vi "WS1050 16 DUT Reliability HD_Cycling Ver1.7.vi"() -> ()   [LabVIEW 2012]
uses:
  Type Defs/WSVCAP SHL I2C DUT Mask Mode Enum.ctl
  <vilib>/Utility/file.llb/Read From Spreadsheet File (DBL).vi
  SubVI/Agilent E363X Series/Agilent E363X Series.lvlib
  SubVI/keithley_2000/Keithley 2000/Keithley 2000.lvlib
  SubVI/2012_Keithley 24XX/Keithley 24XX.lvlib
panel:
  out "VISA resource name out":refnum<visa-resource-name>="GPIB0::3::INSTR"
  out "error out 2":errorcluster={"status"=TRUE, "code"=-63192, "source"="niLvFpga_Open_PXI-7813R.vi"}
  in  "Reg1_Bit Cntrl":string[](array[string])=["01", "02", "04", "08", "10", "20", "40", "80", "03", "06", "0C", "D8", "33", "66", "CC", "07", "0E", "1C", "38", "70", "E0", "0F", "1E", "3C", "78", "F0", "1F", "3E", "7C", "F8", "3F", "7E", "FC", "7F", "FE", "FD", "FB", "F7", "EF", "DF", "BF", "7F", "FC", "F9", "F3", "E7", "CF", "9F", "3F", "F8", "F1", "E3", "C7", "8F", "1F", "F0", "E1", "C3", "87", "0F", "E0", "C1", "83", "07", "C0", "81", "03", "AA", "55", "00"]
  out "date string":string="5/19/2014"
  out "PS1 Out":refnum<visa-resource-name>
  out "Ke2000 Out":refnum<visa-resource-name>="GPIB0::9::INSTR"
  in  "Tab Control":T1(tab)=enum."Data Output"
  in  "Serial Number":string[][](table)=[["DUT", "SN"], ["DUT1", "1"], ["DUT2", "2"], ["DUT3", "3"], ["DUT4", "4"], ["DUT5", "5"], ["DUT6", "6"], ["DUT7", "7"], ["DUT8", "8"], ["DUT9", "9"], ["DUT10", "10"], ["DUT11", "11"], ["DUT12", "12"], ["DUT13", "13"], ["DUT14", "14"], ["DUT15", "15"], ["DUT16", "16"]]
  out "AD7747 Values":string[][](table)
  in  "SPI Clock Rate (Hz)":dbl=5000000.0 caption="Cycle Speed" format="%.1p Hz"
  in  "Lot#":string="3T9BB"
  in  "Wafer#":string="25-EB"
  in  "File Name":string="CYC_3T9BB_25_EB_65C_40V_50DC_BRD3_141107_1"
  in  "TMN DC\\CAP Data Log File Path":path=path "C:/WS1050 16 DUT Data"
  in  "Test Program":string="WS1050 16 DUT Reliability HD_Cycling Ver1.7"
  out "Current Date":string="8/28/2014"
  out "Current Time":string="0950"
  in  "Start Date":string="4/24/2014"
  in  "Start Time":string="1542"
  in  "Comment":string="CYC65C40V"
  in  "OK Button":bool
  in  "Calibration":bool
  in  "Verify CP":bool
  in  "CP Setting":i32(ring) items=["CP OFF", "CP ON", "CP 35V", "CP 40V", "DVA ON", "DVA OFF", "REG1 ON", "REG1 OFF", "REG2 ON", "REG2 OFF", "REG3 ON", "REG3 OFF"]
  in  "Stop Calibration":bool
  in  "Set VDD":dbl=3.7 format="%.3g"
  in  "Command":string[](array[string])=["0702013B3B3B", "070201000000"]
  in  "SPI Clock Rate (Hz)":dbl=1000000.0 caption="Meas Speed" format="%.1p Hz"
  out "AR  Meas(Hz)":dbl
  in  "PS1 Source":refnum<visa-resource-name>="GPIB0::5::INSTR"
  in  "Ke2000":refnum<visa-resource-name>="GPIB0::9::INSTR"
  in  "CP to HD/Cycle":i32(ring)=1 items=["CP HDC 35V", "CP HDC 40.25V", "CP HDC 27.5V", "CP HDC 30.5V", "CP HDC 44V"]
  out "Simulate FPGA":bool
  out "Online":bool
  out "AR Cycling(Hz)":dbl=5000000.0
  in  "Ke2400":refnum<visa-resource-name>="GPIB0::3::INSTR"
  in  "Initialize AD7747":bool
  in  "DUT Mask Mode":T2=enum."All"
  in  "RFFE Slave Address":u8=7 caption="Slave Address" format="0x%02x"
  out "Activity Log":string="05/19/2014 -- 12:24:35.853::WSVCAP::APP::Application Started\n05/19/2014 -- 12:24:37.606::WSVCAP::WSVCAP SHL::WR I2C-REG:0x0A;MASK:0xFFFFFFFFFFFF;C1 DATA:22:22:22:22:22:22:22:22:22:22:22:22:22:22:22:22;C2 DATA:22:22:22:22:22:22:22:22:22:22:22:22:22:22:22:22;C3 DATA:22:22:22:22:22:22:22:22:22:22:22:22:22:22:22:22\r\n05/19/2014 -- 12:24:37.773::WSVCAP::WSVCAP SHL::WR I2C-ST:0,0,4,1\r\n05/19/2014 -- 12:24:37.903::WSVCAP::WSVCAP SHL::RD I2C-BYTES:4;ADD:0x00;MASK:0xFFFFFFFFFFFF\r\n05/19/2014 -- 12:24:38.045::WSVCAP::WSVCAP SHL::RD I2C:C1 DATA:2:2:2:2:2:2:2:2:2:2:2:2:2:2:2:2|A7:A9:AA:82:82:7F:82:81:82:81:83:82:81:82:82:81|46:36:BB:88:44:A3:E9:2B:32:20:ED:25:BB:3D:68:B|2C:6A:EB:A7:22:56:FE:CC:36:82:D7:B0:3B:48:F9:CC;C2 DATA:2:2:2:2:2:2:2:2:2:2:2:2:2:2:2:2|94:94:94:80:80:80:80:80:81:7E:7E:81:80:7E:80:80|47:33:15:82:62:B:E8:1C:D7:C3:7D:41:7C:B7:4C:2A|C4:B4:AE:8:1E:D1:4E:37:11:C0:6F:63:42:9D:63:B5;C3 DATA:2:2:2:2:2:2:2:2:2:2:2:2:2:2:2:2|95:95:95:81:81:7E:81:80:84:7D:80:83:81:7E:7F:80|AB:C4:14:B5:7B:52:DF:C9:79:5D:5F:30:99:31:1E:F4|6E:5C:F7:A8:C3:EB:7B:EF:33:92:89:77:4D:67:75:DD;STATUS:0:0:4:0\r\n05/19/2014 -- 12:24:38.046::WSVCAP::WSVCAP SHL::WR I2C-REG:0x0A;MASK:0xFFFFFFFFFFFF;C1 DATA:22:22:22:22:22:22:22:22:22:22:22:22:22:22:22:22;C2 DATA:22:22:22:22:22:22:22:22:22:22:22:22:22:22:22:22;C3 DATA:22:22:22:22:22:22:22:22:22:22:22:22:22:22:22:22\r\n05/19/2014 -- 12:24:38.089::WSVCAP::WSVCAP SHL::WR I2C-ST:0,0,4,1\r\n05/19/2014 -- 12:24:38.219::WSVCAP::WSVCAP SHL::RD I2C-BYTES:4;ADD:0x00;MASK:0xFFFFFFFFFFFF\r\n05/19/2014 -- 12:24:38.362::WSVCAP::WSVCAP SHL::RD I2C:C1 DATA:2:2:2:2:2:2:2:2:2:2:2:2:2:2:2:2|A7:AB:AA:82:82:82:83:83:82:82:82:82:7F:82:82:81|4B:32:96:83:3E:61:43:17:25:62:AB:4D:A2:40:2E:5|3C:76:2B:B4:EE:E4:A9:1A:AA:A:26:C7:21:2E:87:5B;C2 DATA:2:2:2:2:2:2:2:2:2:2:2:2:2:2:2:2|94:94:94:80:80:80:80:80:80:7F:80:81:80:80:7F:80|4A:32:19:7D:19:6C:79:46:61:7F:4B:B8:A5:30:F3:14|B4:70:A:8C:9C:DC:43:FA:1E:A:C6:21:A:A9:13:F3;C3 DATA:2:2:2:2:2:2:2:2:2:2:2:2:2:2:2:2|95:97:94:81:80:81:82:81:80:7E:81:84:7F:81:80:80|B2:32:D0:A7:9E:4C:AB:D4:EE:D9:F0:82:B7:91:7:FF|C1:91:B6:3D:D8:E:1B:4F:9F:6A:F1:6C:E7:3F:7:BA;STATUS:0:0:4:0\r\n05/19/2014 -- 12:24:38.364::WSVCAP::WSVCAP SHL::WR I2C-REG:0x0A;MASK:0xFFFFFFFFFFFF;C1 DATA:22:22:22:22:22:22:22:22:22:22:22:22:22:22:22:22;C2 DATA:22:22:22:22:22:22:22:22:22:22:22:22:22:22:22:22;C3 DATA:22:22:22:22:22:22:22:22:22:22:22:22:22:22:22:22\r\n05/19/2014 -- 12:24:38.406::WSVCAP::WSVCAP SHL::WR I2C-ST:0,0,4,1\r\n05/19/2014 -- 12:24:38.536::WSVCAP::WSVCAP SHL::RD I2C-BYTES:4;ADD:0x00;MASK:0xFFFFFFFFFFFF\r\n05/19/2014 -- 12:24:38.678::WSVCAP::WSVCAP SHL::RD I2C:C1 DATA:2:2:2:2:2:2:2:2:2:2:2:2:2:2:2:2|A7:A9:AB:82:82:81:82:82:82:82:82:82:82:82:82:81|46:71:4C:87:43:3D:7F:FC:25:4F:8E:54:97:3E:60:8C|AA:F4:1F:B5:CE:43:1F:36:9:87:9C:78:86:5:B6:8E;C2 DATA:2:2:2:2:2:2:2:2:2:2:2:2:2:2:2:2|94:94:94:80:7F:7F:80:80:80:80:80:81:80:80:80:80|49:36:18:7D:6E:C5:E4:3C:81:2E:41:D3:75:71:E3:72|E8:D3:E6:D1:E0:48:AE:D4:54:D:E8:8E:B4:41:68:4;C3 DATA:2:2:2:2:2:2:2:2:2:2:2:2:2:2:2:2|95:95:95:81:7F:7F:81:81:81:81:81:84:81:81:82:81|B3:F5:90:AB:82:69:7B:93:D0:77:E8:D5:E8:8C:84:E8|B9:AC:EE:2B:B6:71:8F:4A:74:31:56:BB:8A:B7:A0:C8;STATUS:0:0:4:0\r\n05/19/2014 -- 12:24:38.681::WSVCAP::WSVCAP SHL::WR I2C-REG:0x0A;MASK:0xFFFFFFFFFFFF;C1 DATA:22:22:22:22:22:22:22:22:22:22:22:22:22:22:22:22;C2 DATA:22:22:22:22:22:22:22:22:22:22:22:22:22:22:22:22;C3 DATA:22:22:22:22:22:22:22:22:22:22:22:22:22:22:22:22\r\n05/19/2014 -- 12:24:38.723::WSVCAP::WSVCAP SHL::WR I2C-ST:0,0,4,1\r\n05/19/2014 -- 12:24:38.854::WSVCAP::WSVCAP SHL::RD I2C-BYTES:4;ADD:0x00;MASK:0xFFFFFFFFFFFF\r\n05/19/2014 -- 12:24:38.996::WSVCAP::WSVCAP SHL::RD I2C:C1 DATA:2:2:2:2:2:2:2:2:2:2:2:2:2:2:2:2|A7:A9:AA:82:82:7F:83:81:82:81:84:82:7F:82:7F:82|43:FB:E:7F:3C:AD:35:35:26:A2:6C:21:4B:3D:8:6|63:9A:E1:F3:95:32:91:42:90:3C:78:1F:5C:D7:5F:D8;C2 DATA:2:2:2:2:2:2:2:2:2:2:2:2:2:2:2:2|94:94:94:80:80:80:80:80:81:80:7E:81:80:7E:7F:80|48:36:18:7F:5E:3D:69:83:DE:AE:A1:9E:31:AE:BB:96|15:A0:44:17:13:FD:CC:C8:6D:B2:EF:A7:C:C7:3B:F;C3 DATA:2:2:2:2:2:2:2:2:2:2:2:2:2:2:2:2|95:96:94:81:81:7E:82:80:84:80:80:84:7F:7E:7D:82|AD:3B:6D:A9:7C:57:9D:F5:7A:96:23:5C:36:2D:ED:5A|CD:46:DB:3B:C7:BD:70:60:33:B8:B:F7:63:A:51:4D;STATUS:0:0:4:0\r\n05/19/2014 -- 12:24:38.998::WSVCAP::WSVCAP SHL::WR I2C-REG:0x0A;MASK:0xFFFFFFFFFFFF;C1 DATA:22:22:22:22:22:22:22:22:22:22:22:22:22:22:22:22;C2 DATA:22:22:22:22:22:22:22:22:22:22:22:22:22:22:22:22;C3 DATA:22:22:22:22:22:22:22:22:22:22:22:22:22:22:22:22\r\n05/19/2014 -- 12:24:39.040::WSVCAP::WSVCAP SHL::WR I2C-ST:0,0,4,1\r\n05/19/2014 -- 12:24:39.170::WSVCAP::WSVCAP SHL::RD I2C-BYTES:4;ADD:0x00;MASK:0xFFFFFFFFFFFF\r\n05/19/2014 -- 12:24:39.311::WSVCAP::WSVCAP SHL::RD I2C:C1 DATA:2:2:2:2:2:2:2:2:2:2:2:2:2:2:2:2|A7:AA:AB:82:82:81:82:81:82:81:82:82:82:82:7F:82|44:F1:90:87:45:44:C8:2C:2C:F1:FC:1B:94:3B:3C:75|4A:49:95:19:99:73:64:3:23:24:F3:A2:5E:7F:C4:B6;C2 DATA:2:2:2:2:2:2:2:2:2:2:2:2:2:2:2:2|94:94:94:80:80:80:80:7F:80:80:7E:80:80:7E:7F:80|4C:36:17:7D:A8:9F:DE:C7:53:6D:8A:F4:41:A5:C6:E0|90:2E:24:C:D9:22:E4:76:3B:40:1D:53:33:B1:3E:4D;C3 DATA:2:2:2:2:2:2:2:2:2:2:2:2:2:2:2:2|95:97:95:81:81:7F:81:80:80:81:7F:82:81:7E:7D:82|AE:2B:A7:AB:CC:CD:A4:38:FD:17:80:F2:92:2D:45:C4|76:E5:D:B9:AD:B5:BA:8D:28:32:9E:42:B7:20:4A:D9;STATUS:0:0:4:0\r\n05/19/2014 -- 12:24:39.313::WSVCAP::WSVCAP SHL::WR I2C-REG:0x0A;MASK:0xFFFFFFFFFFFF;C1 DATA:22:22:22:22:22:22:22:22:22:22:22:22:22:22:22:22;C2 DATA:22:22:22:22:22:22:22:22:22:22:22:22:22:22:22:22;C3 DATA:22:22:22:22:22:22:22:22:22:22:22:22:22:22:22:22\r\n05/19/2014 -- 12:24:39.355::WSVCAP::WSVCAP SHL::WR I2C-ST:0,0,4,1\r\n05/19/2014 -- 12:24:39.486::WSVCAP::WSVCAP SHL::RD I2C-BYTES:4;ADD:0x00;MASK:0xFFFFFFFFFFFF\r\n05/19/2014 -- 12:24:39.628::WSVCAP::WSVCAP SHL::RD I2C:C1 DATA:2:2:2:2:2:2:2:2:2:2:2:2:2:2:2:2|A7:A9:AA:82:82:82:83:82:82:82:82:82:7F:82:7F:82|47:18:E4:87:3E:E7:6:65:25:92:37:38:A8:3E:89:85|7C:A7:7:2B:A3:7A:EC:EF:89:ED:F4:D3:D8:BC:3A:F5;C2 DATA:2:2:2:2:2:2:2:2:2:2:2:2:2:2:2:2|94:94:94:80:7F:80:80:7F:81:80:7E:80:80:80:81:80|49:37:17:80:76:25:6A:F8:DF:55:97:4D:B8:5B:2B:B1|13:E3:9A:3E:1A:2D:4F:B6:DB:E9:61:FA:8B:D6:9:CC;C3 DATA:2:2:2:2:2:2:2:2:2:2:2:2:2:2:2:2|95:95:95:81:7F:80:82:81:84:80:7F:81:80:81:7F:82|AF:93:3B:AF:5B:11:82:E4:7E:C3:2D:72:9:96:D9:A|DB:96:F2:10:5F:64:9A:C6:98:12:27:7D:10:D3:20:D9;STATUS:0:0:4:0\r\n05/19/2014 -- 12:24:40.132::WSVCAP::WSVCAP SHL::CLOSE\r\n"
  in  "C1 Cap DAC":u8=128 caption="B Data In" format="0x%02x"
  in  "C2 Cap DAC":u8=128 caption="B Data In" format="0x%02x"
  in  "C3 Cap DAC":u8=128 caption="B Data In" format="0x%02x"
  out "IDD Brd(uA)":string
  in  "CP to Meas":i32(ring)=1 items=["CP HDC 35V", "CP HDC 40.25V", "CP HDC 27.5V", "CP HDC 30.5V", "CP HDC 44V"]
  in  "25% DC":dbl[](array[numeric])=[1.7e-05, 5e-05] min=0.0 max=0.5 format="%#.0p s"
  in  "50% DC":dbl[](array[numeric])=[3.3e-05, 3.3e-05] min=0.0 max=0.5 format="%#.0p s"
  in  "75% DC":dbl[](array[numeric])=[5e-05, 1.7e-05] min=0.0 max=0.5 format="%#.0p s"
  in  "CP VPI":i32(ring) items=["CP HDC 35V", "CP HDC 40.25V", "CP HDC 27.5V", "CP HDC 30.5V", "CP HDC 44V"]
  in  "Real No. From\nLookup Table":bool
  in  "Control Panel":T3={"Verify Socket"=FALSE, "HD/CYC"=FALSE, "E-CAL"=FALSE, "DVA"=FALSE, "VPI"=TRUE, "VSA"=TRUE, "HS"=TRUE}
  out "Verify Socket":bool
  out "HD/CYC":bool
  out "E-CAL":bool
  out "DVA":bool
  out "VPI":bool
  out "VSA":bool
  out "HS":bool
  in  "Cmd to HD":string="070201383838"
  in  "% Duty Cycle":enum16{"75%_DC", "50%_DC", "25%_DC"}(ring)=enum."25%_DC"
  in  "Set Time (s)\nFor Verify Socket":u32=300
  in  "Freq(Hz)":string="12K"
  in  "Brd #":string="1"
  out "error out":errorcluster
  in  "error in (no error)":errorcluster
  in  "WS1050/51":bool=TRUE
  in  "Test Sequences":i32(ring) items=["C1_C2_C3", "C2_C1_C3", "C3_C2_C1"]
  out "40V_1":string[][](table)
  out "VPI C1":string[][](table)
  out "VPI C3":string[][](table)
  out "NOM IDD OFF(uA)":string
  out "40V_2":string[][](table)
  out "VPI C2":string[][](table)
  out "NOM IDD ON (uA)":string
  out "40V_3":string[][](table)
  out "Total Time":u64
  out "IDD Stdby(uA)":string="2.606990E+0"
  out "EFuse RB T0":string[](array[string])
  out "Current EFuse Read back":string[](array[string])
  in  "Set HD/Cycle \nto Complete":u64=50000000000
  out "No of HD/Cycle\nCompleted":u64
  out "Cycle Count":u64 min=1 max=4 step=1
  out "Loop \ncompleted":i32=1
  out "Previous Time":string="12:20:26 PM"
  out "STATUS":string="Idle...."
  out "IDD_HD/CYC (uA)":string="164.601255E+0"
  in  "stop During HD/Cycles":bool
  in  "stop":bool
  out "Total Delta 2(pF)":string[](array[string])
  out "Total Delta 1(pF)":string[](array[string])
  out "Total Delta 3(pF)":string[](array[string])
  out "% Delta C_T0":string[][](array[string])
  out "% Delta C":string[][](array[string])
  out "EFuse Readback Status":bool[](array[boolean])
  in  "DeltaC Target(pF)_50":dbl=7.375
  out "RB Reg for HD":string[](array[string])
  out "RB Reg for HD/Cycle":string[](array[string])
  in  "DeltaC Target(pF)_51":dbl=5.875
  out "VSA_V1":string[][](table)
  out "VSA_V2":string[][](table)
  out "VSA_V3":string[][](table)
  in  "VSA Voltage(V)":dbl[](array[numeric])=[-10.0, 0.0, 10.0]
  in  "DC_Temp":i32=65
  in  "HD/CYC Temp":i32=65
  in  "Time All ON (s)":u32=120
  in  "Time All OFF (s)":u32=120
  in  "HD_DC (Min)":u64=259200
  out "LPs Count":i32
  in  "X Repeat":i32=100
  out "No LPs to RP":i32
  out "Running Loops":i32=1
  out "TTime Completed":u64=2000
  in  "TTF Completed":u64=50000000000
  in  "HD RP(Min)":dbl=60.0
  in  "CYC RP (X1000)":dbl=10000.0
  out "Min Plot_1":dbl[][](graph) caption="(Y) Multi Plot 2"
  out "Min Plot_2":dbl[][](graph) caption="(Y) Multi Plot 2"
  out "Min Plot_3":dbl[][](graph) caption="(Y) Multi Plot 2"
  in  "Debug":bool
  in  "No of Rows\nFrom Spread Sheet":i32
  in  "Plot Delta Cmin":bool=TRUE
  in  "Plot":T4(ring)
  # "Company:  WiSpry Inc\n20 Fairbanks Ste 198 \nIrvine CA 92618\n\nAuthor:  Andy V Tran\nCreated:  11/24/2014\nLabVIEW 2012 Pro\nTest Program:  WS1050 \n16 DUT HD/Cycle ver1.7\n\n*******************************"
  # "Note for HD during Cycles Setup:\n\n1.  Set HD/Cycle to Completed = 4320 minutes = 72 hours \n(T0 24hrs HD, T2 48hrs HD_Duty Cycle);  Default Setting\n2.  Set Time to Start HD Duty Cycle = 1440 = 24 hours\n3.  Set Time All ON = 120s = 2 minutes\n4.  Set Time All OFF = 120s = 2 minutes\n5.  No of Loops to RP = 3600s/(Time ALL ON(s) + Time ALL + OFF(s))\n6.  X Repeat = X runs\n7.  Set TTF Completed = Repeat X item1 to Stop.\n8.  Stop Test, set TTF Completed = Total Time Completed.\n\nNote for Cycling:\n\n\n\nVersion 1.7 is the latest verision for WS1050 16 DUT test program.\n\n1.  Added Test Sequences"
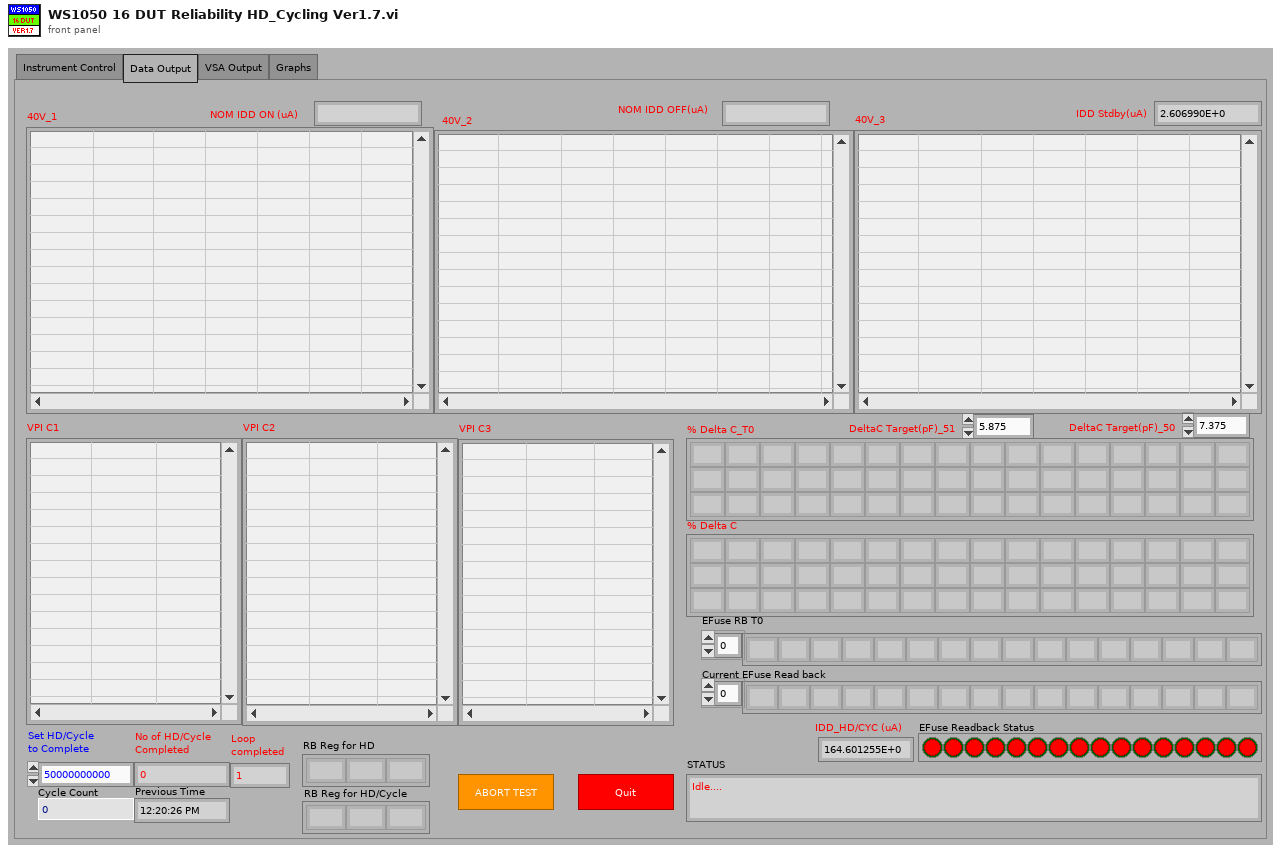
[diagram p1: front panel]
types:
  T1 = enum32{"Instrument Control", "Data Output", "VSA Output", "Graphs"}
  T2 = typedef "WSVCAP SHL I2C DUT Mask Mode Enum.ctl" = enum16{"Custom", "C1", "C2", "C3", "All"}
  T3 = cluster{"Verify Socket":bool, "HD/CYC":bool, "E-CAL":bool, "DVA":bool, "VPI":bool, "VSA":bool, "HS":bool}
  T4 = enum16{"DUT ALL", "DUT 01", "DUT 02", "DUT 03", "DUT 04", "DUT 05", "DUT 06", "DUT 07", "DUT 08", "DUT 09", "DUT 10", "DUT 11", "DUT 12", "DUT 13", "DUT 14", "DUT 15", "DUT 16"}
  T5 = typedef "WSVCAP SHL Core System Cluster.ctl" = cluster{"Settings":T6, "FPGA Resource":tag, "Online":bool, "I2C Wait Ticks":u32, "SPI Wait Ticks":u32, "RFFE Wait Ticks":u32}
  T6 = typedef "WSVCAP SHL I2C Settings Cluster.ctl" = cluster{"FPGA Resource Name":string, "I2C Slave Address":u8, "I2C Clock Rate (Hz)":dbl, "SPI Clock Rate (Hz)":dbl, "RFFE Slave Address":u8, "RFFE Clock Rate (Hz)":dbl, "Simulate FPGA":bool, "C1 Cap DAC Default":u8, "C2 Cap DAC Default":u8, "C3 Cap DAC Default":u8}
  T7 = enum16{"Idle...", "Voltage 1", "Voltage 2", "Voltage 3"}[]
  T8 = cluster{"Test Program ":string, "Comment":string, "Data Out":string, "Data Out":string, "Data Out":string, string, "Data Out":string, "Data Out":string, "string":string, "Freq(Hz)":string, "Brd #":string}
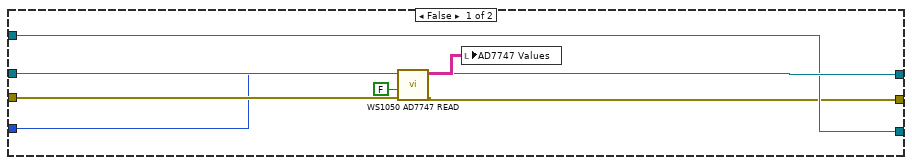
[diagram p9: hidden frame]
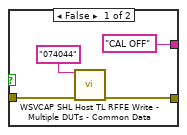
[diagram p10: hidden frame]
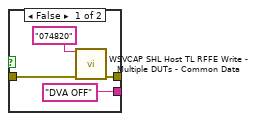
[diagram p11: hidden frame]
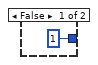
[diagram p12: hidden frame]
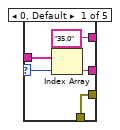
[diagram p13: hidden frame]
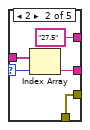
[diagram p14: hidden frame]
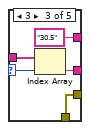
[diagram p15: hidden frame]
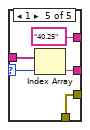
[diagram p16: hidden frame]
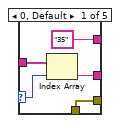
[diagram p17: hidden frame]
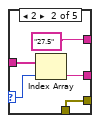
[diagram p18: hidden frame]
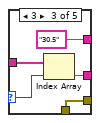
[diagram p19: hidden frame]
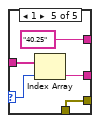
[diagram p20: hidden frame]
diagram:
  w18 = TRUE
  w24 = u16 0 items=["Off", "Moving Filter", "Repeating Filter"] ("Digital Filter (0: Off)")
  w25 = u16 7 items=["3.5 Digits"=4, "4.5 Digits"=5, "5.5 Digits"=6, "6.5 Digits"=7] ("Resolution (7: 6.5 digits)")
  n1 = case shown="True" w18 {
    tunnel: "error in (no error)" -> [w34 w35]
    tunnel: [w34 w42] -> w4
    frame False {
    }
    frame True {
      n2 = call "WSVCAP SHL Host TL Initialize.vi"("error in"=w35) -> ("error out"=w36:errorcluster)  [unwired: 13 in, 1 out]
      n3 = control-ref of="Activity Log"() -> (w38:refnum<vi>)
      n4 = call "ACT LG Activity Log Core.vi"("Display Ref"=w38, "Source"="WSVCAP", "Error In (no error)"=w36) -> ("Error Out"=w37:errorcluster)  [unwired: 11 in, 1 out]
      n5 = call "WSVCAP SHL Host TL Status Manager.vi"("error in"=w37) -> ("System Out"=w43:T5, "error out"=w42:errorcluster)  [unwired: 13 in]
      n6 = Unbundle By Name(w43) -> ("Online"=→"Online":bool, "Settings.Simulate FPGA"=→"Simulate FPGA":bool)
    }
  }
  n7 = case shown="True" TRUE {
    tunnel: w4 -> [w44 w49]
    tunnel: [w45 w48] -> w15
    tunnel: [w44 w47] -> w8
    tunnel: "Ke2400" -> [w45 w46]
    frame False {
    }
    frame True {
      n8 = VISA Write(VISA resource name=w46, write buffer="SOUR:FUNC VOLT;VOLT:MODE FIX;RANG 100;LEV 0.0;:SENS:FUNC \"CURR\";CURR:PROT 60E-3;RANG 100E-3;:OUTP ON", error in (no error)=w49) -> (VISA resource name out=w48:refnum<visa-resource-name>, error out=w47:errorcluster)  [unwired: 1 out]
    }
  }
  n9 = call "Initialize.vi"("VISA resource name"="Ke2000", "error in (no error)"=w4) -> ("VISA resource name out"=w27:refnum<visa-resource-name>, "error out"=w26:errorcluster)  [unwired: 16 in]
  n10 = call "Initialize.vi"("error in (no error)"=w4, "Reset? (T: Yes)"=FALSE, "ID Query? (T: Yes)"=TRUE, "VISA resource name"="PS1 Source") -> ("error out"=w3:errorcluster, "VISA resource name out"=w30:refnum<visa-resource-name>)  [unwired: 6 in]
  n11 = call "Configure DC Current.vi"("VISA resource name"=w27, "Resolution (7: 6.5 digits)"=w25, "error in (no error)"=w26, "Auto Range? (T: Auto)"=FALSE, "Digital Filter (0: Off)"=w24, "Custom Range (0 A)"=1.0) -> ("VISA resource name out"=w22:refnum<visa-resource-name>, "error out"=w5:errorcluster)  [unwired: 12 in]
  n12 = case shown="True" TRUE {
    tunnel: [_ w51] -> w33
    frame False {
    }
    frame True {
      n13 = call-poly <vilib>:"Read From Spreadsheet File.vi"("number of rows (all:-1)"=-1) -> ("all rows"=w51:dbl[][])  [unwired: 6 in, 4 out]
    }
  }
  n14 = Merge Errors(w8, w5, w3) -> (w16:errorcluster)
  n15 = while {
    tunnel: w16 -> [w73]
    tunnel: [w61] -> w12
    tunnel: w33 -> [w79]
    tunnel: w30 -> [w65]
    tunnel: w22 -> [w66]
    tunnel: [w77] -> w21
    tunnel: [w76] -> w20
    tunnel: [FALSE ("stop During HD/Cycles")] -> _
    tunnel: w15 -> [w72]
    tunnel: [w71] -> w13
    tunnel: [FALSE ("stop")] -> w6
    i -> [w74]
    stop <- w80 stop-if-true
    n16 = case shown="0" w74 {
      tunnel: w73 -> [w91 w93]
      tunnel: [w90 w93] -> w68
      tunnel: "RFFE Slave Address" -> [w88 _]
      frame 0 {
        w84 = dbl[][] []
        w83 = "" ("uA")
        w85 = string[][] []
        w86 = string[] [] ("EFuse Read back")
        w92 = u64 0 ("No of HD/Cycle\nCompleted")
        n17 = local write "RB Reg for HD/Cycle"(w86) -> ()
        n18 = local write "Current EFuse Read back"(w86) -> ()
        n19 = local write "EFuse RB T0"(w86) -> ()
        n20 = local write "No of HD/Cycle\nCompleted"(w92) -> ()
        n21 = local write "Cycle Count"(w92) -> ()
        n22 = local write "Total Delta 1(pF)"(w86) -> ()
        n23 = local write "Total Delta 2(pF)"(w86) -> ()
        n24 = local write "Total Delta 3(pF)"(w86) -> ()
        n25 = local write "VPI C2"(w85) -> ()
        n26 = local write "VSA_V3"(w85) -> ()
        n27 = local write "VSA_V1"(w85) -> ()
        n28 = local write "VSA_V2"(w85) -> ()
        n29 = local write "VPI C1"(w85) -> ()
        n30 = local write "VPI C3"(w85) -> ()
        n31 = local write "% Delta C"(w85) -> ()
        n32 = local write "% Delta C_T0"(w85) -> ()
        n33 = local write "40V_2"(w85) -> ()
        n34 = local write "40V_1"(w85) -> ()
        n35 = local write "40V_3"(w85) -> ()
        n36 = local write "NOM IDD OFF(uA)"(w83) -> ()
        n37 = local write "NOM IDD ON (uA)"(w83) -> ()
        n38 = local write "IDD Brd(uA)"(w83) -> ()
        n39 = local write "Min Plot_3"(w84) -> ()
        n40 = local write "Min Plot_1"(w84) -> ()
        n41 = local write "Min Plot_2"(w84) -> ()
        n42 = call "WSVCAP SHL Host TL RFFE Configure.vi"("RFFE Slave Address"=w88, "Clock Rate (Hz)"="SPI Clock Rate (Hz)", "error in"=w91) -> ("Actual Rate (Hz)"=→"AR  Meas(Hz)":dbl, "error out"=w90:errorcluster)  [unwired: 11 in]
      }
      frame 1, Default {
      }
    }
    n43 = while {
      tunnel: ["stop"] -> w70
      tunnel: w68 -> [w113]
      tunnel: [w104] -> w62
      tunnel: w65 -> [w111]
      tunnel: w66 -> [w106]
      tunnel: [w107] -> w64
      tunnel: [w105] -> w63
      tunnel: [w100] -> w59
      tunnel: [w99] -> w58
      tunnel: [w98] -> w57
      tunnel: [w97] -> w56
      tunnel: [w96] -> w55
      tunnel: [w95] -> w54
      tunnel: [w94] -> w53
      stop <- w120 stop-if-true
      # "Set Date & Time to Start Test"
      n44 = case shown="True" "Initialize AD7747" {
        tunnel: w113 -> [w129 w134]
        tunnel: [w129 w130] -> w112
        tunnel: w111 -> [w128 w132]
        tunnel: [w128 w131] -> w110
        frame False {
        }
        frame True {
          w135 = T7 [enum."Voltage 2", enum."Voltage 3", enum."Voltage 1"] items=["Idle...", "Voltage 1", "Voltage 2", "Voltage 3"]
          n45 = for {
            tunnel: w132 -> [w145]
            tunnel: w135 -> [w142] mode=indexing
            tunnel: [w141] -> w131
            shift-right: [w137] -> w133
            shift-left: w134 -> [w146]
            n46 = local read "Set VDD"() -> (w140:dbl)
            n47 = call "E3631A_Voltage Controller.vi"("VISA resource name"=w145, "I_VDD(A)"=0.2, "Channel Controller"=w142, "Voltage 1"=w140, "Voltage 2"=3.3, "error in (no error)"=w146, "Voltage 3"=-3.3) -> ("VISA resource name out"=w141:refnum<visa-resource-name>, "error out"=w136:errorcluster)  [unwired: 7 in]
            n48 = call "Delay T4.vi"("milliseconds to wait"=u32 100, "error in (no error)"=w136) -> ("error out"=w137:errorcluster)  [unwired: 9 in]
          }
          n49 = call "WS1050_AD7747_Init.vi"("error in"=w133) -> ("error out"=w130:errorcluster)  [unwired: 10 in]
        }
      }
      n50 = call "Time_stamp.vi"() -> ("date/time string"=w125:string, "date string"=w127:string)  [unwired: 2 in]
      "Current Date" <- w127
      "Current Time" <- w125
      n51 = Equal?(x=w127, y="Start Date") -> (x = y?=w123:bool)
      n52 = Equal?(x=w125, y="Start Time") -> (x = y?=w122:bool)
      n53 = And(x=w123, y=w122) -> (x .and. y?=w119:bool)
      n54 = Compound Arithmetic op=OR(w119, "OK Button", "stop") -> (w120:bool)
      n55 = case shown="True" "Calibration" {
        tunnel: w112 -> [w175 w193]
        tunnel: [w170 w190] -> w102
        tunnel: w110 -> [w174 w189]
        tunnel: "DUT Mask Mode" -> [w173 w185]
        tunnel: [w174 w184] -> w108
        tunnel: w106 -> [w172 w180]
        tunnel: [w172 w177] -> w105
        frame False {
          n56 = call "WS1050 AD7747 READ.vi"("error in"=w175, "Log (T)"=FALSE, "DUT Mask Mode (All)"=w173) -> ("error out"=w170:errorcluster, "AD7747 Values"=w176:string[][])  [unwired: 7 in]
          n57 = local write "AD7747 Values"(w176) -> ()
        }
        frame True {
          n58 = flat-sequence {
            tunnel: w193 -> [w202]
            tunnel: [w197] -> w192
            tunnel: w189 -> [w201]
            tunnel: [w200] -> w188
            tunnel: w185 -> [w199]
            tunnel: [w199] -> w186
            tunnel: w180 -> [w195]
            tunnel: [w194] -> w179
            tunnel: w192 -> [w226]
            tunnel: [w225] -> w191
            tunnel: w188 -> [w224]
            tunnel: [w224] -> w187
            tunnel: w186 -> [w223]
            tunnel: "C1 Cap DAC" -> [w219]
            tunnel: "C2 Cap DAC" -> [w218]
            tunnel: "C3 Cap DAC" -> [w217]
            tunnel: w179 -> [w216]
            tunnel: [w216] -> w178
            tunnel: w191 -> [w235]
            tunnel: [w238] -> w190
            tunnel: w187 -> [w237]
            tunnel: [w234] -> w184
            tunnel: w178 -> [w233]
            tunnel: [w233] -> w177
            frame #0 {
              w203 = T7 [enum."Voltage 2", enum."Voltage 3", enum."Voltage 1"] items=["Idle...", "Voltage 1", "Voltage 2", "Voltage 3"]
              n59 = for {
                tunnel: w201 -> [w214]
                tunnel: w203 -> [w211] mode=indexing
                tunnel: [w210] -> w200
                shift-right: [w208] -> w196
                shift-left: w202 -> [w215]
                n60 = local read "Set VDD"() -> (w205:dbl)
                n61 = call "E3631A_Voltage Controller.vi"("VISA resource name"=w214, "I_VDD(A)"=0.2, "Channel Controller"=w211, "Voltage 1"=w205, "Voltage 2"=3.3, "error in (no error)"=w215, "Voltage 3"=-3.3) -> ("VISA resource name out"=w210:refnum<visa-resource-name>, "error out"=w207:errorcluster)  [unwired: 7 in]
                n62 = call "Delay T4.vi"("milliseconds to wait"=u32 100, "error in (no error)"=w207) -> ("error out"=w208:errorcluster)  [unwired: 9 in]
              }
              n63 = One Button Dialog(message="Please verify all sockets should be empty...") -> ()  [unwired: 1 in, 1 out]
              n64 = call "Ke2000 Reading MilAmp.vi"("error in (no error)"=w196, "VISA resource name"=w195) -> ("error out"=w197:errorcluster, "uA"=→"IDD Brd(uA)":string, "VISA resource name out"=w194:refnum<visa-resource-name>)  [unwired: 7 in]
            }
            frame #1 {
              # "Calibration Multi-Sockets"
              n65 = call "WS1050 CAPDAC Setting.vi"("DUT Mask Mode (All)"=w223, "error in"=w226, "C3 Cap DAC"=w217, "C2 Cap DAC"=w218, "C1 Cap DAC"=w219) -> ("error out"=w221:errorcluster)  [unwired: 5 in, 1 out]
              n66 = call "WS1050 OFFSET CAL.vi"("error in"=w221, "OFFSET CAL"=TRUE ("Read?")) -> ("error out"=w220:errorcluster)  [unwired: 8 in, 1 out]
              n67 = while {
                tunnel: w220 -> [w232]
                tunnel: [w231] -> w225
                tunnel: w223 -> [w228]
                stop <- "Stop Calibration" stop-if-true
                n68 = call "WS1050 AD7747 READ.vi"("error in"=w232, "Log (T)"=FALSE, "DUT Mask Mode (All)"=w228) -> ("error out"=w231:errorcluster, "AD7747 Values"=→"AD7747 Values":string[][])  [unwired: 7 in]
              }
            }
            frame #2 {
              w236 = T7 [enum."Voltage 2", enum."Voltage 3", enum."Voltage 1"] items=["Idle...", "Voltage 1", "Voltage 2", "Voltage 3"]
              n69 = for {
                tunnel: w237 -> [w250]
                tunnel: w236 -> [w246] mode=indexing
                tunnel: [w245] -> w234
                shift-right: [w241] -> w238
                shift-left: w235 -> [w247]
                n70 = call "E3631A_Voltage Controller.vi"("VISA resource name"=w250, "I_VDD(A)"=0.2, "Channel Controller"=w246, "Voltage 1"=0.0, "Voltage 2"=3.3, "error in (no error)"=w247, "Voltage 3"=-3.3) -> ("VISA resource name out"=w245:refnum<visa-resource-name>, "error out"=w240:errorcluster)  [unwired: 7 in]
                n71 = call "Delay T4.vi"("milliseconds to wait"=u32 100, "error in (no error)"=w240) -> ("error out"=w241:errorcluster)  [unwired: 9 in]
              }
              n72 = One Button Dialog(message="Calibration Completed....") -> ()  [unwired: 1 in, 1 out]
            }
          }
        }
      }
      n73 = call "Control Panel.vi"("error in (no error)"=w102, "Control Panel"="Control Panel") -> ("error out"=w101:errorcluster, "VPI"=w96:bool, "DVA"=w97:bool, "E-CAL"=w98:bool, "VSA"=w95:bool, "HD/CYC"=w99:bool, "HS"=w94:bool, "Verify Socket"=w100:bool)  [unwired: 2 in]
      "Verify Socket" <- w100
      "HS" <- w94
      "VSA" <- w95
      "VPI" <- w96
      "E-CAL" <- w98
      "HD/CYC" <- w99
      "DVA" <- w97
      n74 = case shown="True" "Verify CP" {
        tunnel: [w147 w150] -> w104
        tunnel: w108 -> [w148 w155]
        tunnel: [w148 w153] -> w107
        tunnel: w101 -> [w147 w152]
        frame False {
        }
        frame True {
          w156 = T7 [enum."Voltage 2", enum."Voltage 3", enum."Voltage 1"] items=["Idle...", "Voltage 1", "Voltage 2", "Voltage 3"]
          # "Verify CP"
          n75 = for {
            tunnel: w155 -> [w168]
            tunnel: w156 -> [w165] mode=indexing
            shift-right: [w162] -> w154
            shift-left: w152 -> [w169]
            tunnel: [w160] -> w153
            n76 = local read "Set VDD"() -> (w164:dbl)
            n77 = call "E3631A_Voltage Controller.vi"("VISA resource name"=w168, "Channel Controller"=w165, "Voltage 1"=w164, "Voltage 2"=3.3, "error in (no error)"=w169, "Voltage 3"=-3.3) -> ("VISA resource name out"=w160:refnum<visa-resource-name>, "error out"=w163:errorcluster)  [unwired: 8 in]
            n78 = call "Delay T4.vi"("milliseconds to wait"=u32 100, "error in (no error)"=w163) -> ("error out"=w162:errorcluster)  [unwired: 9 in]
          }
          n79 = Index Array(array=string[] ["074000", "074040", "07476F", "074776", "074800", "074820", "07413B", "074100", "07423B", "074200", "07433B", "074300"], index="CP Setting") -> (element=w157:string)
          n80 = call "WSVCAP SHL Host TL RFFE Write - Multiple DUTs - Common Data.vi"("Data Out"=w157, "error in"=w154) -> ("error out"=w151:errorcluster)  [unwired: 13 in]
          n81 = call "Delay T4.vi"("milliseconds to wait"=u32 10, "error in (no error)"=w151) -> ("error out"=w150:errorcluster)  [unwired: 9 in]
        }
      }
      n82 = Wait Until Next ms Multiple(millisecond multiple=u32 100) -> ()  [unwired: 1 out]
    }
    n83 = case shown="False" w70 {
      tunnel: w62 -> [w306 w1818]
      tunnel: [w290 w1818] -> w61
      tunnel: w79 -> [w307 _]
      tunnel: w64 -> [w305 w1816]
      tunnel: w63 -> [w296 w1817]
      tunnel: [w303 w1817] -> w77
      tunnel: [w300 w1816] -> w76
      tunnel: w72 -> [w293 w1815]
      tunnel: [w289 w1815] -> w71
      tunnel: "RFFE Slave Address" -> [w284 _]
      tunnel: [FALSE ("stop During HD/Cycles") FALSE ("stop During HD/Cycles")] -> w60
      tunnel: w59 -> [w257 _]
      tunnel: w58 -> [w256 _]
      tunnel: w57 -> [w255 _]
      tunnel: w56 -> [w254 _]
      tunnel: w55 -> [w253 _]
      tunnel: w54 -> [w252 _]
      tunnel: w53 -> [w251 _]
      frame False {
        w285 = u64 0 ("Total Completed")
        w263 = u32 100 ("milliseconds to wait")
        w302 = T7 [enum."Voltage 2", enum."Voltage 3", enum."Voltage 1"] items=["Idle...", "Voltage 1", "Voltage 2", "Voltage 3"]
        w304 = T7 [enum."Voltage 2", enum."Voltage 3", enum."Voltage 1"] items=["Idle...", "Voltage 1", "Voltage 2", "Voltage 3"]
        # "DVA"
        # "Verify Socket"
        # "E-CAL"
        # "VSA"
        # "VPI"
        # "HS"
        # "DVA"
        # "HD/CYC"
        n84 = for {
          tunnel: w306 -> [w1813]
          tunnel: w305 -> [w1812]
          tunnel: w304 -> [w1809] mode=indexing
          tunnel: [w1804] -> w298
          tunnel: [w1808] -> w288
          n85 = local read "Set VDD"() -> (w1807:dbl)
          n86 = call "E3631A_Voltage Controller.vi"("VISA resource name"=w1812, "I_VDD(A)"=0.2, "Channel Controller"=w1809, "Voltage 1"=w1807, "Voltage 2"=3.3, "error in (no error)"=w1813, "Voltage 3"=-3.3) -> ("VISA resource name out"=w1808:refnum<visa-resource-name>, "error out"=w1805:errorcluster)  [unwired: 7 in]
          n87 = call "Delay T4.vi"("milliseconds to wait"=u32 100, "error in (no error)"=w1805) -> ("error out"=w1804:errorcluster)  [unwired: 9 in]
        }
        n88 = local write "TTime Completed"(w285) -> ()
        n89 = local write "Total Time"(w285) -> ()
        n90 = call "WSVCAP SHL Host TL RFFE Write - Multiple DUTs - Common Data.vi"("Data Out"="074000", "error in"=w298) -> ("error out"=w299:errorcluster)  [unwired: 13 in]
        n91 = local read "IDD Brd(uA)"() -> (w272:string)
        n92 = call "Delay T4.vi"("milliseconds to wait"=w263, "error in (no error)"=w299) -> ("error out"=w297:errorcluster)  [unwired: 9 in]
        n93 = Number To Fractional String(number="Set VDD", precision (6)=i16 2) -> (F-format string=w278:string)  [unwired: 2 in]
        n94 = call "Ke2000 Reading MilAmp.vi"("error in (no error)"=w297, "VISA resource name"=w296) -> ("error out"=w274:errorcluster, "uA"=w276:string, "VISA resource name out"=w295:refnum<visa-resource-name>)  [unwired: 7 in]
        n95 = call "Substration.vi"("error in (no error)"=w274, "Input2"=w272, "Input1"=w276) -> ("error out"=w273:errorcluster, "In1 - In2"=w275:string)  [unwired: 7 in]
        "IDD Stdby(uA)" <- w275
        n96 = call "WSVCAP SHL Host TL RFFE Write - Multiple DUTs - Common Data.vi"("Data Out"="074040", "error in"=w273) -> ("error out"=w258:errorcluster)  [unwired: 13 in]
        n97 = call "Delay T4.vi"("milliseconds to wait"=w263, "error in (no error)"=w258) -> ("error out"=w282:errorcluster)  [unwired: 9 in]
        n98 = case shown="True" w254 {
          tunnel: w282 -> [w329 w330]
          tunnel: [w328 w331] -> w280
          tunnel: ["DVA OFF" ("Data Out") "DVA ON" ("Data Out")] -> w281
          frame False {
            n99 = call "WSVCAP SHL Host TL RFFE Write - Multiple DUTs - Common Data.vi"("Data Out"="074820", "error in"=w329) -> ("error out"=w328:errorcluster)  [unwired: 13 in]
          }
          frame True {
            n100 = call "WSVCAP SHL Host TL RFFE Write - Multiple DUTs - Common Data.vi"("Data Out"="074800", "error in"=w330) -> ("error out"=w331:errorcluster)  [unwired: 13 in]
          }
        }
        n101 = for {
          N: 16 -> [_]
          tunnel: "Serial Number" -> [w312]
          tunnel: [w310] -> w260 mode=indexing
          i -> [w309]
          n102 = Increment(x=w309) -> (x+1=w308:i32)
          n103 = Index Array(array=w312, index (row)=w308, index (col)=1 ("disabled index (col)")) -> (element=w310:string)
        }
        n104 = case shown="True" w256 {
          tunnel: [1 ("X Repeat") w335] -> w287
          frame False {
          }
          frame True {
            n105 = local read "X Repeat"() -> (w335:i32)
          }
        }
        n106 = Not(x=w251) -> (.not. x?=w259:bool)
        n107 = call "Delay T4.vi"("milliseconds to wait"=w263, "error in (no error)"=w280) -> ("error out"=w267:errorcluster)  [unwired: 9 in]
        n108 = case shown="True" w255 {
          tunnel: w267 -> [w316 w318]
          tunnel: [w313 w317] -> w266
          tunnel: ["CAL OFF" ("Data Out") "CAL ON" ("Data Out")] -> w268
          frame False {
            n109 = call "WSVCAP SHL Host TL RFFE Write - Multiple DUTs - Common Data.vi"("Data Out"="074044", "error in"=w316) -> ("error out"=w313:errorcluster)  [unwired: 13 in]
          }
          frame True {
            n110 = for {
              tunnel: string[] ["074920", "074900"] -> [w325] mode=indexing
              tunnel: w318 -> [w322]
              tunnel: [w321] -> w317
              n111 = call "WSVCAP SHL Host TL RFFE Write - Multiple DUTs - Common Data.vi"("Data Out"=w325, "error in"=w322) -> ("error out"=w324:errorcluster)  [unwired: 13 in]
              n112 = call "Delay T4.vi"("milliseconds to wait"=u32 10, "error in (no error)"=w324) -> ("error out"=w321:errorcluster)  [unwired: 9 in]
            }
          }
        }
        n113 = for {
          N: w287 -> [_]
          tunnel: w307 -> [w372]
          tunnel: [w368] -> w303
          tunnel: [w367] -> w301
          tunnel: w275 -> [w366]
          tunnel: w295 -> [w365]
          tunnel: "TMN DC\\CAP Data Log File Path" -> [w364]
          tunnel: w293 -> [w362]
          tunnel: [w361] -> w291
          tunnel: w288 -> [w360]
          shift-right: [w355] -> _
          shift-left: u64 0 -> [w357]
          tunnel: w256 -> [w354]
          tunnel: w284 -> [w349]
          tunnel: w284 -> [w348]
          tunnel: w281 -> [w347]
          tunnel: w278 -> [w346]
          tunnel: [w345] -> w271
          tunnel: w268 -> [w344]
          tunnel: w266 -> [w343]
          tunnel: w254 -> [w342]
          tunnel: w257 -> [w340]
          tunnel: w253 -> [w339]
          tunnel: w259 -> [w338]
          tunnel: w252 -> [w337]
          tunnel: w260 -> [w336]
          i -> [w353]
          stop <- w341 stop-if-true
          n114 = while {
            tunnel: w372 -> [w592]
            tunnel: w364 -> [w603]
            tunnel: "Lot#" -> [w602]
            tunnel: "Wafer#" -> [w601]
            tunnel: w336 -> [w600]
            tunnel: "Test Program" -> [w599]
            tunnel: w336 -> [w598]
            tunnel: "Comment" -> [w597]
            tunnel: "Lot#" -> [w596]
            tunnel: "Wafer#" -> [w595]
            tunnel: w365 -> [w591]
            tunnel: [w594] -> w368
            tunnel: [w584] -> w367
            tunnel: w366 -> [w590]
            tunnel: w362 -> [w587]
            tunnel: [w586] -> w361
            tunnel: w360 -> [w585]
            tunnel: [w491] -> w351
            tunnel: w353 -> [w529]
            tunnel: [w520] -> w355
            tunnel: w357 -> [w519]
            shift-right: [w518] -> _
            shift-left: u64 0 -> [w412]
            tunnel: [w517] -> w350
            tunnel: w354 -> [w515]
            tunnel: w349 -> [w490]
            tunnel: w348 -> [w488]
            tunnel: w347 -> [w436]
            tunnel: w346 -> [w434]
            tunnel: [w409] -> w345
            tunnel: w344 -> [w416]
            tunnel: w343 -> [w415]
            tunnel: w342 -> [w414]
            tunnel: w340 -> [w406]
            tunnel: w339 -> [w405]
            tunnel: w338 -> [w400]
            tunnel: w337 -> [w394]
            i -> [w516]
            stop <- w530 stop-if-true
            n115 = case shown="4" "CP to HD/Cycle" {
              selector: "CP to HD/Cycle" -> [w607 w612 w617 w622 w626]
              tunnel: string[] ["07476F", "074776", "074765", "074769", "07477B"] -> [w608 w613 w618 w623 w628]
              tunnel: [w606 w611 w616 w621 w627] -> w431
              tunnel: ["35.0" ("Data Out") "27.5" ("Data Out") "30.5" ("Data Out") "44.0" ("Data Out") "40.25" ("Data Out")] -> w430
              tunnel: [w604 w609 w614 w619 w624] -> w429
              tunnel: w415 -> [w604 w609 w614 w619 w624]
              frame 0, Default {
                n116 = Index Array(array=w608, index=w607) -> (element=w606:string)
              }
              frame 2 {
                n117 = Index Array(array=w613, index=w612) -> (element=w611:string)
              }
              frame 3 {
                n118 = Index Array(array=w618, index=w617) -> (element=w616:string)
              }
              frame 4 {
                n119 = Index Array(array=w623, index=w622) -> (element=w621:string)
              }
              frame 1 {
                n120 = Index Array(array=w628, index=w626) -> (element=w627:string)
              }
            }
            n121 = flat-sequence {
              tunnel: [w693] -> w583
              tunnel: [w638] -> w582
              tunnel: w592 -> [w691]
              tunnel: [w690] -> w581
              tunnel: w591 -> [w667]
              tunnel: w590 -> [w689]
              tunnel: [w689] -> w580
              tunnel: [w632] -> w579
              tunnel: [w635] -> w578
              tunnel: w429 -> [w680]
              tunnel: [w647] -> w577
              tunnel: w585 -> [w687]
              tunnel: [w655] -> w584
              tunnel: w529 -> [w685]
              tunnel: w516 -> [w657]
              tunnel: [w657] -> w526
              tunnel: w516 -> [w684]
              tunnel: w515 -> [w682]
              tunnel: [w681] -> w514
              tunnel: [w643] -> w509
              tunnel: [w642] -> w508
              tunnel: [w641] -> w507
              tunnel: [w646] -> w497
              tunnel: [w644] -> w496
              tunnel: w490 -> [w679]
              tunnel: [w679] -> w489
              tunnel: w488 -> [w678]
              tunnel: [w645] -> w475
              tunnel: [w640] -> w449
              tunnel: [w677] -> w437
              tunnel: w431 -> [w675]
              tunnel: [w659] -> w428
              tunnel: [w658] -> w420
              tunnel: w406 -> [w651]
              tunnel: w405 -> [w650]
              tunnel: [w650] -> w404
              tunnel: w400 -> [w649]
              tunnel: [w649] -> w399
              tunnel: w394 -> [w648]
              tunnel: [w648] -> w393
              tunnel: ["WS1050/51"] -> w386
              tunnel: ["Test Sequences"] -> w376
              tunnel: "Real No. From\nLookup Table" -> [w629]
              tunnel: w583 -> [w1016]
              tunnel: [w1012] -> w487
              tunnel: w582 -> [w1015]
              tunnel: w581 -> [w1022]
              tunnel: [w1022] -> w486
              tunnel: w580 -> [w1021]
              tunnel: w579 -> [w1014]
              tunnel: w578 -> [w1013]
              tunnel: [w999] -> w485
              tunnel: [w1021] -> w484
              tunnel: [w1014] -> w483
              tunnel: [w1013] -> w482
              tunnel: w577 -> [w1019]
              tunnel: w526 -> [w1018]
              tunnel: [w1018] -> w481
              tunnel: w514 -> [w1017]
              tunnel: [w1017] -> w480
              tunnel: [w1015] -> w479
              tunnel: w509 -> [w1010]
              tunnel: w508 -> [w1004]
              tunnel: w507 -> [w1002]
              tunnel: [w1007] -> w478
              tunnel: w497 -> [w1009]
              tunnel: w496 -> [w1007]
              tunnel: [w1000] -> w477
              tunnel: w489 -> [w1008]
              tunnel: [w1005] -> w476
              tunnel: w475 -> [w1005]
              tunnel: [w1004] -> w474
              tunnel: w449 -> [w1003]
              tunnel: [w1003] -> w448
              tunnel: [w1002] -> w446
              tunnel: w437 -> [w1006]
              tunnel: [w1001] -> w421
              tunnel: w420 -> [w1001]
              tunnel: w404 -> [w998]
              tunnel: [w998] -> w403
              tunnel: w399 -> [w997]
              tunnel: [w997] -> w398
              tunnel: w393 -> [w996]
              tunnel: [w996] -> w392
              tunnel: w386 -> [w992]
              tunnel: [w992] -> w385
              tunnel: w376 -> [w991]
              tunnel: [w991] -> w375
              tunnel: w487 -> [w1126]
              tunnel: [w1125] -> w473
              tunnel: w486 -> [w1139]
              tunnel: [w1139] -> w470
              tunnel: w485 -> [w1138]
              tunnel: [w1138] -> w468
              tunnel: w484 -> [w1137]
              tunnel: [w1137] -> w466
              tunnel: w483 -> [w1136]
              tunnel: [w1136] -> w464
              tunnel: w482 -> [w1135]
              tunnel: [w1135] -> w462
              tunnel: w481 -> [w1134]
              tunnel: [w1134] -> w460
              tunnel: w480 -> [w1133]
              tunnel: [w1133] -> w458
              tunnel: w479 -> [w1132]
              tunnel: [w1132] -> w456
              tunnel: w478 -> [w1131]
              tunnel: [w1131] -> w454
              tunnel: [w1120] -> w452
              tunnel: w477 -> [w1119]
              tunnel: w476 -> [w1129]
              tunnel: w474 -> [w1127]
              tunnel: w448 -> [w1124]
              tunnel: [w1124] -> w447
              tunnel: w446 -> [w1123]
              tunnel: [w1123] -> w445
              tunnel: [w1121] -> w444
              tunnel: [w1122] -> w422
              tunnel: w421 -> [w1122]
              tunnel: w403 -> [w1118]
              tunnel: [w1118] -> w402
              tunnel: w398 -> [w1117]
              tunnel: [w1117] -> w397
              tunnel: w392 -> [w1116]
              tunnel: [w1116] -> w391
              tunnel: w385 -> [w1115]
              tunnel: [w1115] -> w384
              tunnel: w375 -> [w1114]
              tunnel: [w1114] -> w374
              tunnel: w473 -> [w1212]
              tunnel: [w1211] -> w472
              tunnel: [w1207] -> w471
              tunnel: w470 -> [w1224]
              tunnel: [w1224] -> w469
              tunnel: w468 -> [w1223]
              tunnel: [w1223] -> w467
              tunnel: w466 -> [w1222]
              tunnel: [w1222] -> w465
              tunnel: w464 -> [w1221]
              tunnel: [w1221] -> w463
              tunnel: w462 -> [w1220]
              tunnel: [w1220] -> w461
              tunnel: w460 -> [w1219]
              tunnel: [w1219] -> w459
              tunnel: w458 -> [w1218]
              tunnel: [w1218] -> w457
              tunnel: w456 -> [w1217]
              tunnel: [w1217] -> w455
              tunnel: w454 -> [w1216]
              tunnel: [w1216] -> w453
              tunnel: w452 -> [w1215]
              tunnel: [w1215] -> w451
              tunnel: [w1205] -> w450
              tunnel: w447 -> [w1214]
              tunnel: w445 -> [w1213]
              tunnel: w444 -> [w1206]
              tunnel: [w1210] -> w435
              tunnel: [w1209] -> w423
              tunnel: w422 -> [w1209]
              tunnel: w414 -> [w1208]
              tunnel: [w1208] -> w413
              tunnel: w402 -> [w1204]
              tunnel: [w1204] -> w401
              tunnel: w397 -> [w1203]
              tunnel: [w1203] -> w396
              tunnel: w391 -> [w1202]
              tunnel: [w1202] -> w390
              tunnel: w384 -> [w1201]
              tunnel: [w1201] -> w383
              tunnel: [w1201] -> w381
              tunnel: [w1201] -> w380
              tunnel: w374 -> [w1200]
              tunnel: [w1351] -> w576
              tunnel: [w1317] -> w575
              tunnel: w472 -> [w1355]
              tunnel: w471 -> [w1331]
              tunnel: [w1340] -> w574
              tunnel: [w1331] -> w573
              tunnel: [w1354] -> w572
              tunnel: [w1353] -> w571
              tunnel: w469 -> [w1352]
              tunnel: [w1352] -> w570
              tunnel: w467 -> [w1340]
              tunnel: w465 -> [w1350]
              tunnel: [w1350] -> w569
              tunnel: w463 -> [w1346]
              tunnel: [w1346] -> w568
              tunnel: w461 -> [w1345]
              tunnel: [w1345] -> w567
              tunnel: w459 -> [w1341]
              tunnel: [w1341] -> w525
              tunnel: w457 -> [w1349]
              tunnel: [w1349] -> w513
              tunnel: w455 -> [w1348]
              tunnel: [w1347] -> w510
              tunnel: w453 -> [w1343]
              tunnel: w451 -> [w1339]
              tunnel: [w1344] -> w506
              tunnel: [w1342] -> w505
              tunnel: [w1339] -> w500
              tunnel: w450 -> [w1338]
              tunnel: [w1325] -> w495
              tunnel: [w1324] -> w494
              tunnel: [w1323] -> w493
              tunnel: w435 -> [w1337]
              tunnel: [w1322] -> w424
              tunnel: w423 -> [w1322]
              tunnel: [w1321] -> w419
              tunnel: w413 -> [w1320]
              tunnel: w401 -> [w1315]
              tunnel: w396 -> [w1314]
              tunnel: [w1314] -> w395
              tunnel: w390 -> [w1313]
              tunnel: [w1313] -> w389
              tunnel: w383 -> [w1303]
              tunnel: [w1303] -> w382
              tunnel: w381 -> [w1302]
              tunnel: w380 -> [w1301]
              tunnel: w576 -> [w1568]
              tunnel: [w1568] -> w566
              tunnel: [w1553] -> w565
              tunnel: [w1567] -> w564
              tunnel: w575 -> [w1566]
              tunnel: w574 -> [w1565]
              tunnel: w573 -> [w1564]
              tunnel: [w1565] -> w563
              tunnel: [w1564] -> w562
              tunnel: w572 -> [w1563]
              tunnel: [w1563] -> w561
              tunnel: w571 -> [w1562]
              tunnel: [w1562] -> w560
              tunnel: w570 -> [w1561]
              tunnel: [w1561] -> w559
              tunnel: w569 -> [w1560]
              tunnel: [w1560] -> w558
              tunnel: w568 -> [w1559]
              tunnel: [w1559] -> w557
              tunnel: w567 -> [w1558]
              tunnel: [w1558] -> w556
              tunnel: w587 -> [w1557]
              tunnel: [w1555] -> w555
              tunnel: [w1535] -> w554
              tunnel: [w1536] -> w553
              tunnel: [w1534] -> w552
              tunnel: w525 -> [w1551]
              tunnel: [w1551] -> w524
              tunnel: w513 -> [w1550]
              tunnel: [w1550] -> w512
              tunnel: w510 -> [w1567]
              tunnel: w506 -> [w1548]
              tunnel: w505 -> [w1549]
              tunnel: [w1549] -> w504
              tunnel: [w1548] -> w502
              tunnel: w500 -> [w1547]
              tunnel: [w1547] -> w499
              tunnel: w495 -> [w1533]
              tunnel: w494 -> [w1532]
              tunnel: w493 -> [w1531]
              tunnel: [w1528] -> w492
              tunnel: [w1533] -> w443
              tunnel: [w1532] -> w441
              tunnel: [w1531] -> w439
              tunnel: [w1530] -> w425
              tunnel: w424 -> [w1530]
              tunnel: w419 -> [w1529]
              tunnel: [w1529] -> w418
              tunnel: w395 -> [w1528]
              tunnel: w389 -> [w1527]
              tunnel: w382 -> [w1526]
              tunnel: [w1526] -> w379
              tunnel: w566 -> [w1654]
              tunnel: [w1654] -> w551
              tunnel: w565 -> [w1678]
              tunnel: [w1677] -> w550
              tunnel: w603 -> [w1679]
              tunnel: w602 -> [w1676]
              tunnel: w601 -> [w1675]
              tunnel: w600 -> [w1674]
              tunnel: [w1673] -> w549
              tunnel: w564 -> [w1667]
              tunnel: [w1667] -> w548
              tunnel: w563 -> [w1672]
              tunnel: w562 -> [w1671]
              tunnel: [w1672] -> w547
              tunnel: [w1671] -> w546
              tunnel: [w1662] -> w545
              tunnel: w561 -> [w1670]
              tunnel: [w1670] -> w544
              tunnel: w560 -> [w1669]
              tunnel: [w1669] -> w543
              tunnel: w559 -> [w1666]
              tunnel: [w1668] -> w542
              tunnel: w412 -> [w1665]
              tunnel: [w1664] -> w541
              tunnel: [w1652] -> w540
              tunnel: w558 -> [w1663]
              tunnel: w557 -> [w1661]
              tunnel: w556 -> [w1660]
              tunnel: "File Name" -> [w1659]
              tunnel: w555 -> [w1658]
              tunnel: [w1658] -> w539
              tunnel: w554 -> [w1657]
              tunnel: [w1657] -> w538
              tunnel: [w1656] -> w537
              tunnel: w553 -> [w1656]
              tunnel: w552 -> [w1655]
              tunnel: [w1655] -> w536
              tunnel: [w1650] -> w527
              tunnel: w524 -> [w1651]
              tunnel: [w1651] -> w522
              tunnel: w519 -> [w1649]
              tunnel: w512 -> [w1648]
              tunnel: [w1648] -> w511
              tunnel: w504 -> [w1647]
              tunnel: [w1647] -> w503
              tunnel: w502 -> [w1646]
              tunnel: [w1646] -> w501
              tunnel: w499 -> [w1645]
              tunnel: [w1645] -> w498
              tunnel: w492 -> [w1644]
              tunnel: w443 -> [w1643]
              tunnel: [w1643] -> w442
              tunnel: w441 -> [w1642]
              tunnel: [w1642] -> w440
              tunnel: w439 -> [w1641]
              tunnel: [w1641] -> w438
              tunnel: w428 -> [w1640]
              tunnel: [w1640] -> w427
              tunnel: [w1639] -> w426
              tunnel: w425 -> [w1639]
              tunnel: w418 -> [w1638]
              tunnel: [w1638] -> w417
              tunnel: ["Freq(Hz)"] -> w388
              tunnel: ["Brd #"] -> w387
              tunnel: w379 -> [w1635]
              tunnel: [w1635] -> w378
              tunnel: w551 -> [w1750]
              tunnel: w550 -> [w1749]
              tunnel: w603 -> [w1711]
              tunnel: w599 -> [w1744]
              tunnel: w598 -> [w1747]
              tunnel: w597 -> [w1743]
              tunnel: w596 -> [w1746]
              tunnel: w595 -> [w1742]
              tunnel: w549 -> [w1745]
              tunnel: [w1750] -> w532
              tunnel: [w1748] -> w533
              tunnel: w548 -> [w1740]
              tunnel: [w1740] -> w534
              tunnel: w547 -> [w1739]
              tunnel: w546 -> [w1724]
              tunnel: w545 -> [w1738]
              tunnel: w544 -> [w1737]
              tunnel: w543 -> [w1726]
              tunnel: [w1734] -> w535
              tunnel: w542 -> [w1736]
              tunnel: w541 -> [w1735]
              tunnel: w540 -> [w1734]
              tunnel: "File Name" -> [w1704]
              tunnel: w539 -> [w1733]
              tunnel: [w1733] -> w531
              tunnel: w538 -> [w1732]
              tunnel: w537 -> [w1731]
              tunnel: w536 -> [w1730]
              tunnel: [w1729] -> w528
              tunnel: w527 -> [w1729]
              tunnel: [w1707] -> w523
              tunnel: w522 -> [w1707]
              tunnel: w511 -> [w1728]
              tunnel: w503 -> [w1727]
              tunnel: w501 -> [w1725]
              tunnel: w498 -> [w1723]
              tunnel: w442 -> [w1722]
              tunnel: w440 -> [w1721]
              tunnel: w438 -> [w1720]
              tunnel: w436 -> [w1719]
              tunnel: w416 -> [w1717]
              tunnel: w430 -> [w1716]
              tunnel: w434 -> [w1715]
              tunnel: w427 -> [w1714]
              tunnel: w426 -> [w1713]
              tunnel: w417 -> [w1712]
              tunnel: [w1709] -> w411
              tunnel: [w1700] -> w407
              tunnel: w388 -> [w1699]
              tunnel: w387 -> [w1698]
              tunnel: w378 -> [w1697]
              tunnel: [w1697] -> w377
              tunnel: [w1772] -> w593
              tunnel: [w1773] -> w594
              tunnel: [w1774] -> w491
              tunnel: w535 -> [w1765]
              tunnel: w534 -> [w1773]
              tunnel: w533 -> [w1760]
              tunnel: w532 -> [w1774]
              tunnel: w531 -> [w1767]
              tunnel: [w1767] -> w586
              tunnel: [w1764] -> w520
              tunnel: w528 -> [w1764]
              tunnel: w523 -> [w1766]
              tunnel: [w1766] -> w521
              tunnel: [w1765] -> w518
              tunnel: [w1763] -> w517
              tunnel: [w1759] -> w408
              tunnel: w411 -> [w1758]
              tunnel: w407 -> [w1756]
              tunnel: w377 -> [w1755]
              frame #0 {
                n122 = call "WSVCAP SHL Host TL RFFE Write - Multiple DUTs - Common Data.vi"("Data Out"=w675, "error in"=w680) -> ("error out"=w653:errorcluster)  [unwired: 13 in]
                n123 = Index Array(array=w691, index (row)=w684, index (col)=0 ("disabled index (col)")) -> (element=w683:dbl)
                n124 = for {
                  tunnel: string[] ["0760", "0767", "0768"] -> [w738] mode=indexing
                  tunnel: [w734] -> w664 mode=indexing
                  tunnel: w653 -> [w732]
                  tunnel: [w731] -> w656
                  i -> [w737]
                  n125 = call "Delay T4.vi"("milliseconds to wait"=u32 10, "error in (no error)"=w732) -> ("error out"=w739:errorcluster)  [unwired: 9 in]
                  n126 = call "WSVCAP SHL Host TL RFFE Read - Multiple DUTs - Common Data.vi"("Data Out"=w738, "error in"=w739) -> ("RFFE Data In"=w736:string[], "error out"=w731:errorcluster)  [unwired: 12 in]
                  n127 = Index Array(array=w736, index=w737) -> (element=w733:string)
                  n128 = String Subset(string=w733, offset (0)=0) -> (substring=w734:string)  [unwired: 1 in]
                }
                "RB Reg for HD/Cycle" <- w664
                n129 = call "Delay T4.vi"("milliseconds to wait"=u32 100, "error in (no error)"=w656) -> ("error out"=w670:errorcluster)  [unwired: 9 in]
                n130 = local read "IDD Brd(uA)"() -> (w674:string)
                n131 = call "Ke2000 Reading MilAmp.vi"("error in (no error)"=w670, "VISA resource name"=w667) -> ("error out"=w672:errorcluster, "uA"=w673:string, "VISA resource name out"=w666:refnum<visa-resource-name>)  [unwired: 7 in]
                n132 = call "Substration.vi"("error in (no error)"=w672, "Input2"=w674, "Input1"=w673) -> ("error out"=w669:errorcluster, "In1 - In2"=→"IDD_HD/CYC (uA)":string)  [unwired: 7 in]
                n133 = case shown="False" w682 {
                  tunnel: [w772 w878] -> w693
                  tunnel: [w773 w863] -> w688
                  tunnel: [w771 w880] -> w690
                  tunnel: w669 -> [w767 w867]
                  tunnel: w687 -> [w763 w879]
                  tunnel: [w763 w879] -> w655
                  tunnel: w685 -> [_ w869]
                  tunnel: w683 -> [w764 w864]
                  tunnel: [w769 w865] -> w681
                  tunnel: w657 -> [w750 w861]
                  tunnel: w678 -> [w766 _]
                  tunnel: [w760 "100" ("Data Out")] -> w659
                  tunnel: w651 -> [w748 _]
                  tunnel: w629 -> [w747 w854]
                  frame False {
                    # "Cycles in 1s"
                    n134 = case shown="False" w747 {
                      tunnel: w767 -> [w779 w785]
                      tunnel: w764 -> [w778 w784]
                      tunnel: [w777 w785] -> w762
                      tunnel: w750 -> [w776 _]
                      tunnel: [w775 w784] -> w757
                      tunnel: [u64 1000 ("y") u64 1 ("y")] -> w751
                      frame False {
                        n135 = case shown="8, Default" w776 {
                          tunnel: w778 -> [w781 _]
                          tunnel: [w781 "CYC RP (X1000)"] -> w775
                          tunnel: [w780 w782] -> w777
                          tunnel: w779 -> [w780 w782]
                          frame 0..7 {
                          }
                          frame 8, Default {
                          }
                        }
                      }
                      frame True {
                        # "Read real number\nfrom lookup table"
                      }
                    }
                    n136 = call "WSVCAP SHL Host TL RFFE Configure.vi"("RFFE Slave Address"=w766, "Clock Rate (Hz)"="SPI Clock Rate (Hz)", "error in"=w762) -> ("Actual Rate (Hz)"=→"AR Cycling(Hz)":dbl, "error out"=w758:errorcluster)  [unwired: 11 in]
                    n137 = case shown="\"50%_DC\", Default" "% Duty Cycle" {
                      tunnel: ["75% DC" "50% DC" "25% DC"] -> w755
                      tunnel: ["75" ("Data Out") "50" ("Data Out") "25" ("Data Out")] -> w760
                      tunnel: [w787 w790 w793] -> w759
                      tunnel: w758 -> [w787 w790 w793]
                      frame "75%_DC" {
                      }
                      frame "50%_DC", Default {
                      }
                      frame "25%_DC" {
                      }
                    }
                    n138 = Array Max & Min(array=w755) -> (max value=w754:dbl)  [unwired: 3 out]
                    n139 = Divide(x=1.0, y=w754) -> (x/y=w753:dbl)
                    n140 = To Unsigned Quad Integer(1:w753) -> (0:w752:u64)
                    n141 = Not(x=w748) -> (.not. x?=w749:bool)
                    n142 = case shown="False" w749 {
                      tunnel: [w797 w819] -> w773
                      tunnel: [w800 w818] -> w772
                      tunnel: [u64 1 w817] -> w771
                      tunnel: w759 -> [w798 w816]
                      tunnel: w757 -> [_ w815]
                      tunnel: w755 -> [_ w812]
                      tunnel: w752 -> [_ w811]
                      tunnel: w751 -> [_ w810]
                      tunnel: w750 -> [w796 _]
                      frame False {
                        n143 = case shown="1, Default" w796 {
                          tunnel: w798 -> [w801 w803]
                          tunnel: [w801 w802] -> w797
                          frame 0 {
                          }
                          frame 1, Default {
                            n144 = flat-sequence {
                              tunnel: "Set Time (s)\nFor Verify Socket" -> [w809]
                              tunnel: w803 -> [w806]
                              tunnel: [w806] -> w802
                              frame #0 {
                                n145 = Multiply(x=w809, y=u32 1000) -> (x*y=w808:u32)
                                n146 = Wait (ms)(milliseconds to wait=w808) -> ()  [unwired: 1 out]
                                n147 = local write "STATUS"("Verify Sockets waiting times..." ("STATUS")) -> ()
                              }
                            }
                          }
                        }
                        n148 = local read "stop During HD/Cycles"() -> (w800:bool)
                      }
                      frame True {
                        n149 = while {
                          tunnel: w815 -> [w839]
                          tunnel: [w826] -> w819
                          tunnel: [w831] -> w818
                          tunnel: w816 -> [w837]
                          tunnel: [w825] -> w817
                          tunnel: "Command" -> [w836]
                          tunnel: w812 -> [w835]
                          tunnel: w811 -> [w822]
                          tunnel: w810 -> [w820]
                          i -> [w834]
                          stop <- w830 stop-if-true
                          # "At least 1 second before target"
                          # "Remaining Cycles"
                          # "Target Cycles"
                          # "Cycles in 1s"
                          n150 = To Unsigned Quad Integer(1:w839) -> (0:w838:u64)
                          n151 = case shown="0" w834 {
                            tunnel: [w846 w848] -> w828
                            tunnel: w837 -> [w847 w848]
                            tunnel: w836 -> [w845 _]
                            tunnel: w835 -> [w844 _]
                            frame 0 {
                              n152 = call "WSVCAP SHL Host TL RFFE Write Cycle - Multiple DUTs - Common Data1.vi"("Data Out (Cycle Commands)"=w845, "Post Command Delay"=w844, "error in"=w847) -> ("error out"=w846:errorcluster)  [unwired: 12 in]
                            }
                            frame 1, Default {
                            }
                          }
                          n153 = Multiply(x=w838, y=w820) -> (x*y=w825:u64)
                          n154 = call "WSVCAP SHL Host TL SPI_RFFE Query Cycle Count.vi"("error in"=w828) -> ("Cycle Count"=w824:u64, "error out"=w833:errorcluster)  [unwired: 13 in]
                          "Cycle Count" <- w824
                          n155 = Subtract(x=w825, y=w824) -> (x-y=w823:u64)
                          n156 = Greater Or Equal?(x=w824, y=w825) -> (x >= y?=w832:bool)
                          n157 = local read "stop During HD/Cycles"() -> (w831:bool)
                          n158 = Greater?(x=w823, y=w822) -> (0:w821:bool)
                          n159 = case shown="True" w832 {
                            tunnel: [w850 w853] -> w827
                            tunnel: w833 -> [w850 w852]
                            tunnel: [FALSE TRUE] -> w829
                            frame False {
                            }
                            frame True {
                              n160 = call "WSVCAP SHL Host TL RFFE Stop Write Cycle.vi"("error in"=w852) -> ("error out"=w853:errorcluster)  [unwired: 14 in]
                            }
                          }
                          n161 = Or(x=w829, y=w831) -> (x .or. y?=w830:bool)
                          n162 = case shown="True" w821 {
                            tunnel: w827 -> [w840 w843]
                            tunnel: [w840 w842] -> w826
                            frame False {
                            }
                            frame True {
                              n163 = call "MISC Wait with Data Flow.vi"("Error In (no error)"=w843, "Wait Time (500ms)"=u32 50) -> ("Error Out"=w842:errorcluster)  [unwired: 7 in, 2 out]
                            }
                          }
                        }
                        n164 = local write "STATUS"("Parts are Cycling...." ("STATUS")) -> ()
                      }
                    }
                    n165 = local read "HD/CYC Temp"() -> (w768:i32)
                    n166 = Number To Engineering String(4:w768) -> (0:w769:string)  [unwired: 3 in]
                  }
                  frame True {
                    n167 = case shown="False" w854 {
                      tunnel: w869 -> [w886 _]
                      tunnel: [w885 w898] -> w868
                      tunnel: w867 -> [w884 w899]
                      tunnel: [w883 w899] -> w866
                      tunnel: w864 -> [w882 w898]
                      tunnel: w861 -> [w881 _]
                      frame False {
                        n168 = case shown="0" w886 {
                          tunnel: [w889 w896] -> w885
                          tunnel: w884 -> [w891 w897]
                          tunnel: [w890 w897] -> w883
                          tunnel: w882 -> [w888 _]
                          tunnel: w881 -> [w887 _]
                          frame 0 {
                            n169 = case shown="15, Default" w887 {
                              tunnel: [w892 "HD RP(Min)"] -> w889
                              tunnel: w891 -> [w893 w895]
                              tunnel: [w893 w895] -> w890
                              tunnel: w888 -> [w892 _]
                              frame 0..14 {
                              }
                              frame 15, Default {
                              }
                            }
                          }
                          frame 1, Default {
                            n170 = local read "HD RP(Min)"() -> (w896:dbl)
                          }
                        }
                      }
                      frame True {
                      }
                    }
                    n171 = flat-sequence {
                      tunnel: [w973] -> w874
                      tunnel: w866 -> [w979]
                      frame #0 {
                        n172 = call "WSVCAP SHL Host TL RFFE Write - Multiple DUTs - Common Data.vi"("Data Out"="Cmd to HD", "error in"=w979) -> ("error out"=w978:errorcluster)  [unwired: 13 in]
                        n173 = call "Delay T4.vi"("milliseconds to wait"=u32 50, "error in (no error)"=w978) -> ("error out"=w975:errorcluster)  [unwired: 9 in]
                        n174 = for {
                          tunnel: string[] ["0761", "0762", "0763"] -> [w990] mode=indexing
                          tunnel: [w986] -> w974 mode=indexing
                          shift-right: [w983] -> w973
                          shift-left: w975 -> [w989]
                          i -> [w988]
                          n175 = call "WSVCAP SHL Host TL RFFE Read - Multiple DUTs - Common Data.vi"("Data Out"=w990, "error in"=w989) -> ("RFFE Data In"=w985:string[], "error out"=w982:errorcluster)  [unwired: 12 in]
                          n176 = Index Array(array=w985, index=w988) -> (element=w984:string)
                          n177 = call "Delay T4.vi"("milliseconds to wait"=u32 10, "error in (no error)"=w982) -> ("error out"=w983:errorcluster)  [unwired: 9 in]
                          n178 = String Subset(string=w984, offset (0)=0) -> (substring=w986:string)  [unwired: 1 in]
                        }
                        "RB Reg for HD" <- w974
                      }
                    }
                    n179 = local read "No of HD/Cycle\nCompleted"() -> (w870:u64)
                    n180 = Greater?(x="HD_DC (Min)", y=w870) -> (0:w871:bool)
                    n181 = case shown="True" w871 {
                      tunnel: [_ w906] -> w876
                      tunnel: [w901 w905] -> w875
                      tunnel: w874 -> [w901 w904]
                      tunnel: w868 -> [w900 w903]
                      tunnel: [w900 w902] -> w873
                      frame False {
                      }
                      frame True {
                        n182 = flat-sequence {
                          tunnel: [w911] -> w906
                          tunnel: [w910] -> w905
                          tunnel: w904 -> [w909]
                          tunnel: w903 -> [w907]
                          tunnel: [w907] -> w902
                          frame #0 {
                            # "HD"
                            n183 = Multiply(x=1000.0, y=w907) -> (x*y=w914:dbl)
                            n184 = Multiply(x=60.0, y=w914) -> (x*y=w912:dbl)
                            n185 = local write "STATUS"("Parts are Holding Down..." ("STATUS")) -> ()
                            n186 = event shown="[0] Timeout" {
                              selector: _ -> [_ _]
                              dyn-events: _ -> [_ _]
                              timeout: w912 -> [_ _]
                              tunnel: ["stop During HD/Cycles" TRUE ("stop During HD/Cycles")] -> w911
                              tunnel: w909 -> [w916 w918]
                              tunnel: [w916 w918] -> w910
                              event Timeout {
                                n187 = event-data() -> ()  [unwired: 1 in, 2 out]
                              }
                              event "stop During HD/Cycles": Value Change {
                                n188 = event-data() -> ()  [unwired: 1 in, 2 out]
                              }
                            }
                          }
                        }
                      }
                    }
                    n189 = Greater Or Equal?(x=w870, y="HD_DC (Min)") -> (x >= y?=w877:bool)
                    n190 = To Unsigned Quad Integer(1:w868) -> (0:w880:u64)
                    n191 = Add(x="Time All OFF (s)", y="Time All ON (s)") -> (x+y=w856:u32)
                    n192 = To Double Precision Float(number=w856) -> (double precision float=w855:dbl)
                    n193 = Divide(x=w855, y=60.0) -> (x/y=w857:dbl)
                    n194 = case shown="False" w877 {
                      tunnel: [w922 w935] -> w878
                      tunnel: [w923 w927] -> w863
                      tunnel: w875 -> [w923 w934]
                      tunnel: w876 -> [w922 w933]
                      tunnel: w873 -> [_ w932]
                      tunnel: [w921 w930] -> w865
                      tunnel: w857 -> [_ w924]
                      frame False {
                        n195 = Number To Engineering String(4:"HD/CYC Temp") -> (0:w921:string)  [unwired: 3 in]
                      }
                      frame True {
                        n196 = Divide(x=w932, y=w924) -> (x/y=w931:dbl)
                        n197 = call "WSVCAP SHL Host TL RFFE Write - Multiple DUTs - Common Data.vi"("Data Out"="070201000000", "error in"=w934) -> ("error out"=w937:errorcluster)  [unwired: 13 in]
                        n198 = Round To Nearest(number=w931) -> (nearest integer value=w926:dbl)
                        n199 = call "Delay T4.vi"("milliseconds to wait"=u32 50, "error in (no error)"=w937) -> ("error out"=w928:errorcluster)  [unwired: 9 in]
                        n200 = To Long Integer(number=w926) -> (32bit integer=w925:i32)
                        "No LPs to RP" <- w925
                        n201 = for {
                          N: w925 -> [_]
                          tunnel: w933 -> [w952]
                          tunnel: [w951] -> w935
                          tunnel: w928 -> [w940]
                          tunnel: [w939] -> w927
                          i -> [w950]
                          stop <- w951 stop-if-true
                          n202 = Increment(x=w950) -> (x+1=→"LPs Count":i32)
                          n203 = call "WSVCAP SHL Host TL RFFE Write - Multiple DUTs - Common Data.vi"("Data Out"="074776", "error in"=w940) -> ("error out"=w958:errorcluster)  [unwired: 13 in]
                          n204 = call "Delay T4.vi"("milliseconds to wait"=u32 1, "error in (no error)"=w958) -> ("error out"=w957:errorcluster)  [unwired: 9 in]
                          n205 = local read "CP to HD/Cycle"() -> (w942:i32)
                          n206 = call "WSVCAP SHL Host TL RFFE Write - Multiple DUTs - Common Data.vi"("Data Out"="070201000000", "error in"=w943) -> ("error out"=w954:errorcluster)  [unwired: 13 in]
                          n207 = call "WSVCAP SHL Host TL RFFE Write - Multiple DUTs - Common Data.vi"("Data Out"="0702013B3B3B", "error in"=w957) -> ("error out"=w947:errorcluster)  [unwired: 13 in]
                          n208 = flat-sequence {
                            tunnel: w954 -> [w966]
                            tunnel: [w964] -> w939
                            frame #0 {
                              n209 = local read "Time All OFF (s)"() -> (w961:u32)
                              n210 = local write "STATUS"("Now HD OFF Time..." ("STATUS")) -> ()
                              n211 = Multiply(x=w961, y=u32 1000) -> (x*y=w963:u32)
                              n212 = call "Delay T4.vi"("milliseconds to wait"=w963, "error in (no error)"=w966) -> ("error out"=w964:errorcluster)  [unwired: 9 in]
                            }
                          }
                          n213 = call "Delay T4.vi"("milliseconds to wait"=u32 1, "error in (no error)"=w947) -> ("error out"=w945:errorcluster)  [unwired: 9 in]
                          n214 = Index Array(array=string[] ["07476F", "074776", "074765", "074769", "07477B"], index=w942) -> (element=w948:string)
                          n215 = call "WSVCAP SHL Host TL RFFE Write - Multiple DUTs - Common Data.vi"("Data Out"=w948, "error in"=w945) -> ("error out"=w944:errorcluster)  [unwired: 13 in]
                          n216 = flat-sequence {
                            tunnel: [w971] -> w943
                            tunnel: w944 -> [w967]
                            frame #0 {
                              n217 = local read "Time All ON (s)"() -> (w968:u32)
                              n218 = local write "STATUS"("Now HD ON Time..." ("STATUS")) -> ()
                              n219 = Multiply(x=w968, y=u32 1000) -> (x*y=w970:u32)
                              n220 = call "Delay T4.vi"("milliseconds to wait"=w970, "error in (no error)"=w967) -> ("error out"=w971:errorcluster)  [unwired: 9 in]
                            }
                          }
                          n221 = Unbundle By Name(w939) -> ("status"=w953:bool)
                          n222 = Or(x=w953, y=w952) -> (x .or. y?=w951:bool)
                        }
                        n223 = Number To Engineering String(4:"DC_Temp") -> (0:w930:string)  [unwired: 3 in]
                      }
                    }
                  }
                }
                n224 = case shown="4" "CP to Meas" {
                  selector: "CP to Meas" -> [w709 w714 w719 w724 w728]
                  tunnel: string[] ["07476F", "074776", "074765", "074769", "07477B"] -> [w710 w715 w720 w725 w730]
                  tunnel: [w708 w713 w718 w723 w729] -> w662
                  tunnel: [w707 w712 w717 w722 w727] -> w652
                  tunnel: w661 -> [w707 w712 w717 w722 w727]
                  tunnel: ["35" ("Data Out") "27.5" ("Data Out") "30.5" ("Data Out") "44.0" ("Data Out") "40.25" ("Data Out")] -> w658
                  frame 0, Default {
                    n225 = Index Array(array=w710, index=w709) -> (element=w708:string)
                  }
                  frame 2 {
                    n226 = Index Array(array=w715, index=w714) -> (element=w713:string)
                  }
                  frame 3 {
                    n227 = Index Array(array=w720, index=w719) -> (element=w718:string)
                  }
                  frame 4 {
                    n228 = Index Array(array=w725, index=w724) -> (element=w723:string)
                  }
                  frame 1 {
                    n229 = Index Array(array=w730, index=w728) -> (element=w729:string)
                  }
                }
                n230 = call "WSVCAP SHL Host TL RFFE Write - Multiple DUTs - Common Data.vi"("Data Out"=w662, "error in"=w652) -> ("error out"=w676:errorcluster)  [unwired: 13 in]
                n231 = flat-sequence {
                  tunnel: w688 -> [w746]
                  tunnel: [w746] -> w661
                  frame #0 {
                    w742 = "0" ("NOM IDD OFF(uA)")
                    w743 = string[] []
                    w744 = string[][] []
                    n232 = To Long Integer(number=0.0 ("No of Loops to RP")) -> (32bit integer=w741:i32)
                    n233 = local write "LPs Count"(w741) -> ()
                    n234 = local write "No LPs to RP"(w741) -> ()
                    n235 = local write "NOM IDD ON (uA)"(w742) -> ()
                    n236 = local write "Current EFuse Read back"(w743) -> ()
                    n237 = local write "RB Reg for HD"(w743) -> ()
                    n238 = local write "RB Reg for HD/Cycle"(w743) -> ()
                    n239 = local write "NOM IDD OFF(uA)"(w742) -> ()
                    n240 = local write "Total Delta 1(pF)"(w743) -> ()
                    n241 = local write "Total Delta 2(pF)"(w743) -> ()
                    n242 = local write "Total Delta 3(pF)"(w743) -> ()
                    n243 = local write "VSA_V3"(w744) -> ()
                    n244 = local write "VSA_V1"(w744) -> ()
                    n245 = local write "VSA_V2"(w744) -> ()
                    n246 = local write "VPI C1"(w744) -> ()
                    n247 = local write "VPI C2"(w744) -> ()
                    n248 = local write "VPI C3"(w744) -> ()
                    n249 = local write "% Delta C"(w744) -> ()
                    n250 = local write "40V_3"(w744) -> ()
                    n251 = local write "40V_2"(w744) -> ()
                    n252 = local write "40V_1"(w744) -> ()
                  }
                }
                n253 = call "Delay T4.vi"("milliseconds to wait"=u32 50, "error in (no error)"=w676) -> ("error out"=w654:errorcluster)  [unwired: 9 in]
                n254 = for {
                  tunnel: [w705] -> w633 mode=indexing
                  tunnel: w666 -> [w703]
                  tunnel: w654 -> [w702]
                  tunnel: [w696] -> w638
                  tunnel: string[] ["0702013B3B3B", "070201000000"] -> [w695] mode=indexing
                  tunnel: [w694] -> w631
                  n255 = call "WSVCAP SHL Host TL RFFE Write - Multiple DUTs - Common Data.vi"("Data Out"=w695, "error in"=w702) -> ("error out"=w699:errorcluster)  [unwired: 13 in]
                  n256 = call "Delay T4.vi"("milliseconds to wait"=u32 100, "error in (no error)"=w699) -> ("error out"=w700:errorcluster)  [unwired: 9 in]
                  n257 = local read "IDD Brd(uA)"() -> (w704:string)
                  n258 = call "Ke2000 Reading MilAmp.vi"("error in (no error)"=w700, "VISA resource name"=w703) -> ("error out"=w698:errorcluster, "uA"=w697:string, "VISA resource name out"=w696:refnum<visa-resource-name>)  [unwired: 7 in]
                  n259 = call "Substration.vi"("error in (no error)"=w698, "Input2"=w704, "Input1"=w697) -> ("error out"=w694:errorcluster, "In1 - In2"=w705:string)  [unwired: 7 in]
                }
                n260 = Index Array(array=w633, index=0) -> (element=w635:string)
                n261 = Index Array(array=w633, index=1) -> (element=w632:string)
                n262 = call "Multi Dut Cmd Setting.vi"("error in (no error)"=w631, "Test Seq"="Test Sequences", "WS1050/51"="WS1050/51") -> ("error out"=w647:errorcluster, "Cmd 3"=w641:string[], "Name 3"=w640:string[], "Name Header"=w644:string[], "Cmd 2"=w642:string[], "Name 2"=w645:string[], "Cmd 1"=w643:string[], "Name 1"=w646:string[])  [unwired: 1 in]
                n263 = local read "SPI Clock Rate (Hz)"() -> (w677:dbl)
              }
              frame #1 {
                n264 = call "WSVCAP SHL Host TL RFFE Configure.vi"("RFFE Slave Address"=w1008, "Clock Rate (Hz)"=w1006, "error in"=w1019) -> ("Actual Rate (Hz)"=w1020:dbl, "error out"=w994:errorcluster)  [unwired: 11 in]
                n265 = local write "AR  Meas(Hz)"(w1020) -> ()
                n266 = Array Size(array=w1009) -> (size(s)=w1023:i32)
                n267 = call "Delay T4.vi"("milliseconds to wait"=u32 10, "error in (no error)"=w994) -> ("error out"=w995:errorcluster)  [unwired: 9 in]
                n268 = case shown="2" w991 {
                  tunnel: w1023 -> [w1031 w1061 w1091]
                  tunnel: w1016 -> [w1030 w1060 w1090]
                  tunnel: [w1029 w1059 w1089] -> w1012
                  tunnel: [w1028 w1058 w1088] -> w1011
                  tunnel: w1010 -> [w1027 w1057 w1087]
                  tunnel: w1009 -> [w1026 w1056 w1086]
                  tunnel: [w1025 w1055 w1085] -> w1000
                  tunnel: w995 -> [w1024 w1054 w1084]
                  frame 0, Default {
                    n269 = for {
                      N: w1031 -> [_]
                      tunnel: w1027 -> [w1049]
                      tunnel: w1030 -> [w1047]
                      tunnel: [w1046] -> w1029
                      tunnel: [w1042] -> w1028 mode=indexing
                      tunnel: w1026 -> [w1044]
                      tunnel: w1024 -> [w1032]
                      tunnel: [w1034] -> w1025
                      i -> [w1041]
                      stop <- w1046 stop-if-true
                      n270 = Index Array(array=w1049, index=w1041) -> (element=w1045:string)
                      n271 = Index Array(array=w1044, index=w1041) -> (element=w1043:string)
                      n272 = local write "STATUS"(w1043) -> ()
                      n273 = call "WSVCAP SHL Host TL RFFE Write - Multiple DUTs - Common Data.vi"("Data Out"=w1045, "error in"=w1032) -> ("error out"=w1036:errorcluster)  [unwired: 13 in]
                      n274 = call "Delay T4.vi"("milliseconds to wait"=u32 10, "error in (no error)"=w1036) -> ("error out"=w1040:errorcluster)  [unwired: 9 in]
                      n275 = call "WS1050 AD7747 READ.vi"("error in"=w1040, "Log (T)"=FALSE, "DUT Mask Mode (All)"=WSVCAP_SHL_I2C_DUT_Mask_Mode_Enum."C1") -> ("error out"=w1038:errorcluster, "AD7747 Values"=w1039:string[][])  [unwired: 7 in]
                      n276 = for {
                        tunnel: w1039 -> [w1052] mode=indexing
                        tunnel: w1038 -> [w1053]
                        tunnel: [w1053] -> w1034
                        tunnel: [w1050] -> w1042 mode=indexing
                        n277 = Index Array(array=w1052, index=1) -> (element=w1050:string)
                      }
                      n278 = Unbundle By Name(w1034) -> ("status"=w1048:bool)
                      n279 = Or(x=w1048, y=w1047) -> (x .or. y?=w1046:bool)
                    }
                  }
                  frame 1 {
                    n280 = for {
                      N: w1061 -> [_]
                      tunnel: w1057 -> [w1079]
                      tunnel: w1060 -> [w1077]
                      tunnel: [w1076] -> w1059
                      tunnel: [w1072] -> w1058 mode=indexing
                      tunnel: w1056 -> [w1074]
                      tunnel: w1054 -> [w1062]
                      tunnel: [w1064] -> w1055
                      i -> [w1071]
                      stop <- w1076 stop-if-true
                      n281 = Index Array(array=w1079, index=w1071) -> (element=w1075:string)
                      n282 = Index Array(array=w1074, index=w1071) -> (element=w1073:string)
                      n283 = local write "STATUS"(w1073) -> ()
                      n284 = call "WSVCAP SHL Host TL RFFE Write - Multiple DUTs - Common Data.vi"("Data Out"=w1075, "error in"=w1062) -> ("error out"=w1066:errorcluster)  [unwired: 13 in]
                      n285 = call "Delay T4.vi"("milliseconds to wait"=u32 10, "error in (no error)"=w1066) -> ("error out"=w1070:errorcluster)  [unwired: 9 in]
                      n286 = call "WS1050 AD7747 READ.vi"("error in"=w1070, "Log (T)"=FALSE, "DUT Mask Mode (All)"=WSVCAP_SHL_I2C_DUT_Mask_Mode_Enum."C2") -> ("error out"=w1068:errorcluster, "AD7747 Values"=w1069:string[][])  [unwired: 7 in]
                      n287 = for {
                        tunnel: w1069 -> [w1082] mode=indexing
                        tunnel: w1068 -> [w1083]
                        tunnel: [w1083] -> w1064
                        tunnel: [w1080] -> w1072 mode=indexing
                        n288 = Index Array(array=w1082, index=3) -> (element=w1080:string)
                      }
                      n289 = Unbundle By Name(w1064) -> ("status"=w1078:bool)
                      n290 = Or(x=w1078, y=w1077) -> (x .or. y?=w1076:bool)
                    }
                  }
                  frame 2 {
                    n291 = for {
                      N: w1091 -> [_]
                      tunnel: w1087 -> [w1109]
                      tunnel: w1090 -> [w1107]
                      tunnel: [w1106] -> w1089
                      tunnel: [w1102] -> w1088 mode=indexing
                      tunnel: w1086 -> [w1104]
                      tunnel: w1084 -> [w1092]
                      tunnel: [w1094] -> w1085
                      i -> [w1101]
                      stop <- w1106 stop-if-true
                      n292 = Index Array(array=w1109, index=w1101) -> (element=w1105:string)
                      n293 = Index Array(array=w1104, index=w1101) -> (element=w1103:string)
                      n294 = local write "STATUS"(w1103) -> ()
                      n295 = call "WSVCAP SHL Host TL RFFE Write - Multiple DUTs - Common Data.vi"("Data Out"=w1105, "error in"=w1092) -> ("error out"=w1096:errorcluster)  [unwired: 13 in]
                      n296 = call "Delay T4.vi"("milliseconds to wait"=u32 10, "error in (no error)"=w1096) -> ("error out"=w1100:errorcluster)  [unwired: 9 in]
                      n297 = call "WS1050 AD7747 READ.vi"("error in"=w1100, "Log (T)"=FALSE, "DUT Mask Mode (All)"=WSVCAP_SHL_I2C_DUT_Mask_Mode_Enum."C3") -> ("error out"=w1098:errorcluster, "AD7747 Values"=w1099:string[][])  [unwired: 7 in]
                      n298 = for {
                        tunnel: w1099 -> [w1112] mode=indexing
                        tunnel: w1098 -> [w1113]
                        tunnel: [w1113] -> w1094
                        tunnel: [w1110] -> w1102 mode=indexing
                        n299 = Index Array(array=w1112, index=5) -> (element=w1110:string)
                      }
                      n300 = Unbundle By Name(w1094) -> ("status"=w1108:bool)
                      n301 = Or(x=w1108, y=w1107) -> (x .or. y?=w1106:bool)
                    }
                  }
                }
                n302 = Transpose 2D Array(2D array=w1011) -> (transposed array=w999:string[][])
                "40V_1" <- w999
                "NOM IDD ON (uA)" <- w1014
                "NOM IDD OFF(uA)" <- w1013
              }
              frame #2 {
                n303 = Array Size(array=w1129) -> (size(s)=w1130:i32)
                n304 = case shown="0, 2, Default" w1114 {
                  tunnel: w1130 -> [w1147 w1177]
                  tunnel: w1129 -> [w1146 w1176]
                  tunnel: [w1145 w1175] -> w1128
                  tunnel: w1127 -> [w1144 w1174]
                  tunnel: w1126 -> [w1143 w1173]
                  tunnel: [w1142 w1172] -> w1125
                  tunnel: [w1141 w1171] -> w1121
                  tunnel: w1119 -> [w1140 w1170]
                  frame 0, 2, Default {
                    n305 = for {
                      N: w1147 -> [_]
                      tunnel: w1144 -> [w1165]
                      tunnel: w1143 -> [w1163]
                      tunnel: [w1162] -> w1142
                      tunnel: [w1158] -> w1145 mode=indexing
                      tunnel: w1146 -> [w1160]
                      tunnel: w1140 -> [w1148]
                      tunnel: [w1150] -> w1141
                      i -> [w1157]
                      stop <- w1162 stop-if-true
                      n306 = Index Array(array=w1165, index=w1157) -> (element=w1161:string)
                      n307 = Index Array(array=w1160, index=w1157) -> (element=w1159:string)
                      n308 = call "WSVCAP SHL Host TL RFFE Write - Multiple DUTs - Common Data.vi"("Data Out"=w1161, "error in"=w1148) -> ("error out"=w1152:errorcluster)  [unwired: 13 in]
                      n309 = local write "STATUS"(w1159) -> ()
                      n310 = call "Delay T4.vi"("milliseconds to wait"=u32 10, "error in (no error)"=w1152) -> ("error out"=w1156:errorcluster)  [unwired: 9 in]
                      n311 = call "WS1050 AD7747 READ.vi"("error in"=w1156, "Log (T)"=FALSE, "DUT Mask Mode (All)"=WSVCAP_SHL_I2C_DUT_Mask_Mode_Enum."C2") -> ("error out"=w1154:errorcluster, "AD7747 Values"=w1155:string[][])  [unwired: 7 in]
                      n312 = for {
                        tunnel: w1155 -> [w1168] mode=indexing
                        tunnel: w1154 -> [w1169]
                        tunnel: [w1169] -> w1150
                        tunnel: [w1166] -> w1158 mode=indexing
                        n313 = Index Array(array=w1168, index=3) -> (element=w1166:string)
                      }
                      n314 = Unbundle By Name(w1150) -> ("status"=w1164:bool)
                      n315 = Or(x=w1164, y=w1163) -> (x .or. y?=w1162:bool)
                    }
                  }
                  frame 1 {
                    n316 = for {
                      N: w1177 -> [_]
                      tunnel: w1174 -> [w1195]
                      tunnel: w1173 -> [w1193]
                      tunnel: [w1192] -> w1172
                      tunnel: [w1188] -> w1175 mode=indexing
                      tunnel: w1176 -> [w1190]
                      tunnel: w1170 -> [w1178]
                      tunnel: [w1180] -> w1171
                      i -> [w1187]
                      stop <- w1192 stop-if-true
                      n317 = Index Array(array=w1195, index=w1187) -> (element=w1191:string)
                      n318 = Index Array(array=w1190, index=w1187) -> (element=w1189:string)
                      n319 = call "WSVCAP SHL Host TL RFFE Write - Multiple DUTs - Common Data.vi"("Data Out"=w1191, "error in"=w1178) -> ("error out"=w1182:errorcluster)  [unwired: 13 in]
                      n320 = local write "STATUS"(w1189) -> ()
                      n321 = call "Delay T4.vi"("milliseconds to wait"=u32 10, "error in (no error)"=w1182) -> ("error out"=w1186:errorcluster)  [unwired: 9 in]
                      n322 = call "WS1050 AD7747 READ.vi"("error in"=w1186, "Log (T)"=FALSE, "DUT Mask Mode (All)"=WSVCAP_SHL_I2C_DUT_Mask_Mode_Enum."C1") -> ("error out"=w1184:errorcluster, "AD7747 Values"=w1185:string[][])  [unwired: 7 in]
                      n323 = for {
                        tunnel: w1185 -> [w1198] mode=indexing
                        tunnel: w1184 -> [w1199]
                        tunnel: [w1199] -> w1180
                        tunnel: [w1196] -> w1188 mode=indexing
                        n324 = Index Array(array=w1198, index=1) -> (element=w1196:string)
                      }
                      n325 = Unbundle By Name(w1180) -> ("status"=w1194:bool)
                      n326 = Or(x=w1194, y=w1193) -> (x .or. y?=w1192:bool)
                    }
                  }
                }
                n327 = Transpose 2D Array(2D array=w1128) -> (transposed array=w1120:string[][])
                "40V_2" <- w1120
              }
              frame #3 {
                n328 = case shown="True" w1201 {
                  tunnel: w1214 -> [_ w1237]
                  tunnel: w1213 -> [_ w1236]
                  tunnel: w1212 -> [w1229 w1231]
                  tunnel: [w1229 w1235] -> w1211
                  tunnel: [string[][] [] w1234] -> w1207
                  tunnel: w1206 -> [w1227 w1233]
                  tunnel: [w1227 w1232] -> w1205
                  tunnel: w1200 -> [_ w1230]
                  frame False {
                  }
                  frame True {
                    n329 = Array Size(array=w1237) -> (size(s)=w1238:i32)
                    n330 = case shown="2" w1230 {
                      tunnel: w1238 -> [w1247 w1278]
                      tunnel: w1237 -> [w1246 w1277]
                      tunnel: w1236 -> [w1245 w1276]
                      tunnel: [w1244 w1275] -> w1235
                      tunnel: [w1242 w1273] -> w1234
                      tunnel: w1233 -> [w1241 w1272]
                      tunnel: [w1240 w1271] -> w1232
                      tunnel: w1231 -> [w1239 w1270]
                      frame 0, 1, Default {
                        n331 = for {
                          N: w1247 -> [_]
                          tunnel: w1245 -> [w1265]
                          tunnel: w1239 -> [w1263]
                          tunnel: [w1262] -> w1244
                          tunnel: [w1258] -> w1243 mode=indexing
                          tunnel: w1246 -> [w1260]
                          tunnel: w1241 -> [w1248]
                          tunnel: [w1250] -> w1240
                          i -> [w1257]
                          stop <- w1262 stop-if-true
                          n332 = Index Array(array=w1265, index=w1257) -> (element=w1261:string)
                          n333 = Index Array(array=w1260, index=w1257) -> (element=w1259:string)
                          n334 = local write "STATUS"(w1259) -> ()
                          n335 = call "WSVCAP SHL Host TL RFFE Write - Multiple DUTs - Common Data.vi"("Data Out"=w1261, "error in"=w1248) -> ("error out"=w1252:errorcluster)  [unwired: 13 in]
                          n336 = call "Delay T4.vi"("milliseconds to wait"=u32 10, "error in (no error)"=w1252) -> ("error out"=w1256:errorcluster)  [unwired: 9 in]
                          n337 = call "WS1050 AD7747 READ.vi"("error in"=w1256, "Log (T)"=FALSE, "DUT Mask Mode (All)"=WSVCAP_SHL_I2C_DUT_Mask_Mode_Enum."C3") -> ("error out"=w1254:errorcluster, "AD7747 Values"=w1255:string[][])  [unwired: 7 in]
                          n338 = for {
                            tunnel: w1255 -> [w1268] mode=indexing
                            tunnel: w1254 -> [w1269]
                            tunnel: [w1269] -> w1250
                            tunnel: [w1266] -> w1258 mode=indexing
                            n339 = Index Array(array=w1268, index=5) -> (element=w1266:string)
                          }
                          n340 = Unbundle By Name(w1250) -> ("status"=w1264:bool)
                          n341 = Or(x=w1264, y=w1263) -> (x .or. y?=w1262:bool)
                        }
                        n342 = Transpose 2D Array(2D array=w1243) -> (transposed array=w1242:string[][])
                      }
                      frame 2 {
                        n343 = for {
                          N: w1278 -> [_]
                          tunnel: w1276 -> [w1296]
                          tunnel: w1270 -> [w1294]
                          tunnel: [w1293] -> w1275
                          tunnel: [w1289] -> w1274 mode=indexing
                          tunnel: w1277 -> [w1291]
                          tunnel: w1272 -> [w1279]
                          tunnel: [w1281] -> w1271
                          i -> [w1288]
                          stop <- w1293 stop-if-true
                          n344 = Index Array(array=w1296, index=w1288) -> (element=w1292:string)
                          n345 = Index Array(array=w1291, index=w1288) -> (element=w1290:string)
                          n346 = local write "STATUS"(w1290) -> ()
                          n347 = call "WSVCAP SHL Host TL RFFE Write - Multiple DUTs - Common Data.vi"("Data Out"=w1292, "error in"=w1279) -> ("error out"=w1283:errorcluster)  [unwired: 13 in]
                          n348 = call "Delay T4.vi"("milliseconds to wait"=u32 10, "error in (no error)"=w1283) -> ("error out"=w1287:errorcluster)  [unwired: 9 in]
                          n349 = call "WS1050 AD7747 READ.vi"("error in"=w1287, "Log (T)"=FALSE, "DUT Mask Mode (All)"=WSVCAP_SHL_I2C_DUT_Mask_Mode_Enum."C1") -> ("error out"=w1285:errorcluster, "AD7747 Values"=w1286:string[][])  [unwired: 7 in]
                          n350 = for {
                            tunnel: w1286 -> [w1299] mode=indexing
                            tunnel: w1285 -> [w1300]
                            tunnel: [w1300] -> w1281
                            tunnel: [w1297] -> w1289 mode=indexing
                            n351 = Index Array(array=w1299, index=1) -> (element=w1297:string)
                          }
                          n352 = Unbundle By Name(w1281) -> ("status"=w1295:bool)
                          n353 = Or(x=w1295, y=w1294) -> (x .or. y?=w1293:bool)
                        }
                        n354 = Transpose 2D Array(2D array=w1274) -> (transposed array=w1273:string[][])
                      }
                    }
                  }
                }
                "40V_3" <- w1207
                n355 = case shown="False" w1201 {
                  tunnel: ["DeltaC Target(pF)_51" "DeltaC Target(pF)_50"] -> w1210
                  frame False {
                  }
                  frame True {
                  }
                }
              }
              frame #4 {
                # "VPI Testing @ 35V"
                n356 = call "WS1050 Delta C Calculation.vi"("WS1050/51"=w1303, "error in (no error)"=w1338, "DCap Target(pF)"=w1337, "Input"=w1340) -> ("error out"=w1335:errorcluster, "Total Bank Delta C(pF)"=w1328:string[], "% Bank DeltaC"=w1332:string[])  [unwired: 3 in, 2 out]
                n357 = call "WS1050 Delta C Calculation.vi"("WS1050/51"=w1302, "error in (no error)"=w1338, "DCap Target(pF)"=w1337, "Input"=w1339) -> ("error out"=w1336:errorcluster, "Total Bank Delta C(pF)"=w1327:string[], "% Bank DeltaC"=w1330:string[])  [unwired: 3 in, 2 out]
                n358 = call "WS1050 Delta C Calculation.vi"("WS1050/51"=w1301, "error in (no error)"=w1338, "DCap Target(pF)"=w1337, "Input"=w1331) -> ("error out"=w1334:errorcluster, "Total Bank Delta C(pF)"=w1326:string[], "% Bank DeltaC"=w1329:string[])  [unwired: 3 in, 2 out]
                n359 = Merge Errors(w1335, w1336, w1334) -> (w1333:errorcluster)
                n360 = case shown="1, Default" w1341 {
                  tunnel: w1333 -> [w1369 w1377]
                  tunnel: [w1369 w1377] -> w1305
                  tunnel: w1332 -> [w1365 w1373]
                  tunnel: w1330 -> [w1364 w1372]
                  tunnel: w1329 -> [w1363 w1371]
                  tunnel: w1328 -> [w1368 w1376]
                  tunnel: [w1368 w1376] -> w1325
                  tunnel: w1327 -> [w1367 w1375]
                  tunnel: [w1367 w1375] -> w1324
                  tunnel: w1326 -> [w1366 w1374]
                  tunnel: [w1366 w1374] -> w1323
                  frame 0 {
                    n361 = Build Array(w1365, w1364, w1363) -> (→"% Delta C_T0":string[][])
                  }
                  frame 1, Default {
                    n362 = Build Array(w1373, w1372, w1371) -> (→"% Delta C":string[][])
                  }
                }
                "Total Delta 1(pF)" <- w1325
                "Total Delta 2(pF)" <- w1324
                "Total Delta 3(pF)" <- w1323
                n363 = call "Multi Dut Cmd VPI Setting.vi"("error in (no error)"=w1305, "WS1050/51"=w1303) -> ("error out"=w1304:errorcluster, "Cmd VPI C3"=w1306:string[], "VPI_C3"=w1310:string[], "Name Header VPI"=w1309:string[], "Cmd VPI C2"=w1307:string[], "VPI_C2"=w1311:string[], "Cmd VPI C1"=w1308:string[], "VPI_C1"=w1312:string[])  [unwired: 2 in]
                n364 = case shown="True" w1315 {
                  tunnel: w1355 -> [w1379 w1407]
                  tunnel: [w1378 w1388] -> w1319
                  tunnel: [w1381 w1409] -> w1354
                  tunnel: [w1381 w1395] -> w1353
                  tunnel: [w1379 w1393] -> w1351
                  tunnel: w1348 -> [w1382 w1408]
                  tunnel: [w1382 w1408] -> w1347
                  tunnel: w1308 -> [_ w1406]
                  tunnel: w1307 -> [_ w1400]
                  tunnel: w1306 -> [_ w1396]
                  tunnel: [w1381 w1405] -> w1344
                  tunnel: w1312 -> [_ w1403]
                  tunnel: w1311 -> [_ w1401]
                  tunnel: w1310 -> [_ w1397]
                  tunnel: ["NA" ("string") w1392] -> w1321
                  tunnel: w1304 -> [w1378 w1384]
                  tunnel: w1303 -> [_ w1383]
                  frame False {
                    w1381 = string[][] []
                  }
                  frame True {
                    # "Set CP to 35V"
                    n365 = flat-sequence {
                      tunnel: [w1469] -> w1389
                      tunnel: w1384 -> [w1467]
                      tunnel: [w1474] -> w1392
                      tunnel: w1389 -> [w1473]
                      tunnel: [w1472] -> w1387
                      frame #0 {
                        n366 = call "WSVCAP SHL Host TL RFFE Write - Multiple DUTs - Common Data.vi"("Data Out"="074820", "error in"=w1467) -> ("error out"=w1470:errorcluster)  [unwired: 13 in]
                        n367 = call "Delay T4.vi"("milliseconds to wait"=u32 10, "error in (no error)"=w1470) -> ("error out"=w1469:errorcluster)  [unwired: 9 in]
                      }
                      frame #1 {
                        n368 = case shown="4" "CP VPI" {
                          selector: "CP VPI" -> [w1482 w1487 w1492 w1497 w1501]
                          tunnel: string[] ["07476F", "074776", "074765", "074769", "07477B"] -> [w1483 w1488 w1493 w1498 w1503]
                          tunnel: [w1481 w1486 w1491 w1496 w1502] -> w1477
                          tunnel: [w1479 w1484 w1489 w1494 w1499] -> w1476
                          tunnel: ["35" ("string") "27.5" ("string") "30.5" ("string") "44.0" ("string") "40.25" ("string")] -> w1474
                          tunnel: w1473 -> [w1479 w1484 w1489 w1494 w1499]
                          frame 0, Default {
                            n369 = Index Array(array=w1483, index=w1482) -> (element=w1481:string)
                          }
                          frame 2 {
                            n370 = Index Array(array=w1488, index=w1487) -> (element=w1486:string)
                          }
                          frame 3 {
                            n371 = Index Array(array=w1493, index=w1492) -> (element=w1491:string)
                          }
                          frame 4 {
                            n372 = Index Array(array=w1498, index=w1497) -> (element=w1496:string)
                          }
                          frame 1 {
                            n373 = Index Array(array=w1503, index=w1501) -> (element=w1502:string)
                          }
                        }
                        n374 = call "WSVCAP SHL Host TL RFFE Write - Multiple DUTs - Common Data.vi"("Data Out"=w1477, "error in"=w1476) -> ("error out"=w1472:errorcluster)  [unwired: 13 in]
                      }
                    }
                    n375 = Array Size(array=w1403) -> (size(s)=w1410:i32)
                    n376 = call "Delay T4.vi"("milliseconds to wait"=u32 50, "error in (no error)"=w1387) -> ("error out"=w1386:errorcluster)  [unwired: 9 in]
                    n377 = for {
                      N: w1410 -> [_]
                      tunnel: w1406 -> [w1521]
                      tunnel: w1407 -> [w1519]
                      tunnel: [w1518] -> w1399
                      tunnel: [w1516] -> w1404 mode=indexing
                      tunnel: w1403 -> [w1515]
                      tunnel: w1386 -> [w1504]
                      tunnel: [w1506] -> w1391
                      i -> [w1514]
                      stop <- w1518 stop-if-true
                      n378 = Index Array(array=w1521, index=w1514) -> (element=w1517:string)
                      n379 = Index Array(array=w1515, index=w1514) -> (element=w1513:string)
                      n380 = call "WSVCAP SHL Host TL RFFE Write - Multiple DUTs - Common Data.vi"("Data Out"=w1517, "error in"=w1504) -> ("error out"=w1512:errorcluster)  [unwired: 13 in]
                      n381 = local write "STATUS"(w1513) -> ()
                      n382 = call "Delay T4.vi"("milliseconds to wait"=u32 10, "error in (no error)"=w1512) -> ("error out"=w1508:errorcluster)  [unwired: 9 in]
                      n383 = call "WS1050 AD7747 READ.vi"("error in"=w1508, "Log (T)"=FALSE, "DUT Mask Mode (All)"=WSVCAP_SHL_I2C_DUT_Mask_Mode_Enum."C1") -> ("error out"=w1510:errorcluster, "AD7747 Values"=w1509:string[][])  [unwired: 7 in]
                      n384 = for {
                        tunnel: [w1524] -> w1516 mode=indexing
                        tunnel: w1510 -> [w1523]
                        tunnel: [w1523] -> w1506
                        tunnel: w1509 -> [w1522] mode=indexing
                        n385 = Index Array(array=w1522, index=1) -> (element=w1524:string)
                      }
                      n386 = Unbundle By Name(w1506) -> ("status"=w1520:bool)
                      n387 = Or(x=w1520, y=w1519) -> (x .or. y?=w1518:bool)
                    }
                    n388 = Transpose 2D Array(2D array=w1404) -> (transposed array=w1409:string[][])
                    "VPI C1" <- w1409
                    n389 = Array Size(array=w1401) -> (size(s)=w1402:i32)
                    n390 = for {
                      N: w1402 -> [_]
                      tunnel: w1400 -> [w1462]
                      tunnel: w1399 -> [w1460]
                      tunnel: [w1459] -> w1394
                      tunnel: [w1457] -> w1398 mode=indexing
                      tunnel: w1401 -> [w1456]
                      tunnel: w1391 -> [w1445]
                      tunnel: [w1447] -> w1390
                      i -> [w1455]
                      stop <- w1459 stop-if-true
                      n391 = Index Array(array=w1462, index=w1455) -> (element=w1458:string)
                      n392 = Index Array(array=w1456, index=w1455) -> (element=w1454:string)
                      n393 = call "WSVCAP SHL Host TL RFFE Write - Multiple DUTs - Common Data.vi"("Data Out"=w1458, "error in"=w1445) -> ("error out"=w1453:errorcluster)  [unwired: 13 in]
                      n394 = local write "STATUS"(w1454) -> ()
                      n395 = call "Delay T4.vi"("milliseconds to wait"=u32 10, "error in (no error)"=w1453) -> ("error out"=w1449:errorcluster)  [unwired: 9 in]
                      n396 = call "WS1050 AD7747 READ.vi"("error in"=w1449, "Log (T)"=FALSE, "DUT Mask Mode (All)"=WSVCAP_SHL_I2C_DUT_Mask_Mode_Enum."C2") -> ("error out"=w1451:errorcluster, "AD7747 Values"=w1450:string[][])  [unwired: 7 in]
                      n397 = for {
                        tunnel: [w1465] -> w1457 mode=indexing
                        tunnel: w1451 -> [w1464]
                        tunnel: [w1464] -> w1447
                        tunnel: w1450 -> [w1463] mode=indexing
                        n398 = Index Array(array=w1463, index=3) -> (element=w1465:string)
                      }
                      n399 = Unbundle By Name(w1447) -> ("status"=w1461:bool)
                      n400 = Or(x=w1461, y=w1460) -> (x .or. y?=w1459:bool)
                    }
                    n401 = Transpose 2D Array(2D array=w1398) -> (transposed array=w1405:string[][])
                    "VPI C2" <- w1405
                    n402 = case shown="True" w1383 {
                      tunnel: w1397 -> [_ w1421]
                      tunnel: w1396 -> [_ w1420]
                      tunnel: [string[][] [] w1418] -> w1395
                      tunnel: w1394 -> [w1413 w1417]
                      tunnel: [w1413 w1416] -> w1393
                      tunnel: w1390 -> [w1412 w1415]
                      tunnel: [w1412 w1414] -> w1388
                      frame False {
                      }
                      frame True {
                        n403 = Array Size(array=w1421) -> (size(s)=w1422:i32)
                        n404 = for {
                          N: w1422 -> [_]
                          tunnel: w1420 -> [w1440]
                          tunnel: w1417 -> [w1438]
                          tunnel: [w1437] -> w1416
                          tunnel: [w1435] -> w1419 mode=indexing
                          tunnel: w1421 -> [w1434]
                          tunnel: w1415 -> [w1423]
                          tunnel: [w1425] -> w1414
                          i -> [w1433]
                          stop <- w1437 stop-if-true
                          n405 = Index Array(array=w1440, index=w1433) -> (element=w1436:string)
                          n406 = Index Array(array=w1434, index=w1433) -> (element=w1432:string)
                          n407 = call "WSVCAP SHL Host TL RFFE Write - Multiple DUTs - Common Data.vi"("Data Out"=w1436, "error in"=w1423) -> ("error out"=w1431:errorcluster)  [unwired: 13 in]
                          n408 = local write "STATUS"(w1432) -> ()
                          n409 = call "Delay T4.vi"("milliseconds to wait"=u32 10, "error in (no error)"=w1431) -> ("error out"=w1427:errorcluster)  [unwired: 9 in]
                          n410 = call "WS1050 AD7747 READ.vi"("error in"=w1427, "Log (T)"=FALSE, "DUT Mask Mode (All)"=WSVCAP_SHL_I2C_DUT_Mask_Mode_Enum."C3") -> ("error out"=w1429:errorcluster, "AD7747 Values"=w1428:string[][])  [unwired: 7 in]
                          n411 = for {
                            tunnel: [w1443] -> w1435 mode=indexing
                            tunnel: w1429 -> [w1442]
                            tunnel: [w1442] -> w1425
                            tunnel: w1428 -> [w1441] mode=indexing
                            n412 = Index Array(array=w1441, index=5) -> (element=w1443:string)
                          }
                          n413 = Unbundle By Name(w1425) -> ("status"=w1439:bool)
                          n414 = Or(x=w1439, y=w1438) -> (x .or. y?=w1437:bool)
                        }
                        n415 = Transpose 2D Array(2D array=w1419) -> (transposed array=w1418:string[][])
                      }
                    }
                    "VPI C3" <- w1395
                  }
                }
                n416 = Insert Into Array(array=w1343, new element=w1309) -> (w1342:string[])  [unwired: 1 in]
                n417 = case shown="False" w1320 {
                  tunnel: w1319 -> [w1356 w1360]
                  tunnel: [w1357 w1359] -> w1318
                  frame False {
                    n418 = call "WSVCAP SHL Host TL RFFE Write - Multiple DUTs - Common Data.vi"("Data Out"="074820", "error in"=w1356) -> ("error out"=w1357:errorcluster)  [unwired: 13 in]
                  }
                  frame True {
                    n419 = call "WSVCAP SHL Host TL RFFE Write - Multiple DUTs - Common Data.vi"("Data Out"="074800", "error in"=w1360) -> ("error out"=w1359:errorcluster)  [unwired: 13 in]
                  }
                }
                n420 = call "Delay T4.vi"("milliseconds to wait"=u32 50, "error in (no error)"=w1318) -> ("error out"=w1317:errorcluster)  [unwired: 9 in]
              }
              frame #5 {
                # "VSA Testing"
                n421 = case shown="True" w1527 {
                  tunnel: w1566 -> [w1580 w1582]
                  tunnel: [w1580 w1581] -> w1540
                  tunnel: [w1579 w1588] -> w1556
                  tunnel: w1557 -> [w1579 w1587]
                  tunnel: [w1577 w1585] -> w1545
                  tunnel: [w1577 w1584] -> w1542
                  tunnel: [w1577 w1583] -> w1539
                  tunnel: [string[][] [] w1586] -> w1546
                  frame False {
                    w1577 = string[][] []
                  }
                  frame True {
                    n422 = for {
                      tunnel: "VSA Voltage(V)" -> [w1612] mode=indexing
                      tunnel: [w1616] -> w1588
                      tunnel: w1587 -> [w1614]
                      tunnel: [w1613] -> w1585 mode=indexing
                      tunnel: [w1600] -> w1584 mode=indexing
                      tunnel: [w1609] -> w1586 mode=indexing
                      tunnel: [w1594] -> w1583 mode=indexing
                      tunnel: w1582 -> [w1593]
                      tunnel: [w1592] -> w1581
                      w1591 = FALSE ("Log (T)")
                      w1608 = u16 0 items=["Voltage", "Current"] ("Source Mode  (0: Voltage)")
                      n423 = call "Configure Output.vi"("Source Mode  (0: Voltage)"=w1608, "error in (no error)"=w1593, "Compliance  Level (0.1)"=0.1, "Output Level (0)"=w1612, "VISA resource name"=w1614) -> ("error out"=w1620:errorcluster, "VISA resource name out"=w1618:refnum<visa-resource-name>)  [unwired: 5 in]
                      n424 = Number To Fractional String(number=w1612) -> (F-format string=w1611:string)  [unwired: 3 in]
                      n425 = call "Enable Output.vi"("error in (no error)"=w1620, "Enable Output (T: Enable)"=TRUE, "VISA resource name"=w1618) -> ("error out"=w1621:errorcluster, "VISA resource name out"=w1616:refnum<visa-resource-name>)  [unwired: 7 in]
                      n426 = call "Delay T4.vi"("milliseconds to wait"=u32 10, "error in (no error)"=w1621) -> ("error out"=w1607:errorcluster)  [unwired: 9 in]
                      n427 = call "WS1050 AD7747 READ.vi"("error in"=w1607, "Log (T)"=w1591, "DUT Mask Mode (All)"=WSVCAP_SHL_I2C_DUT_Mask_Mode_Enum."C1") -> ("error out"=w1604:errorcluster, "AD7747 Values"=w1606:string[][])  [unwired: 7 in]
                      n428 = for {
                        tunnel: w1606 -> [w1632] mode=indexing
                        tunnel: [w1633] -> w1613 mode=indexing
                        tunnel: w1604 -> [w1631]
                        tunnel: [w1631] -> w1603
                        n429 = Index Array(array=w1632, index=1) -> (element=w1633:string)
                      }
                      n430 = for {
                        N: 16 -> [_]
                        tunnel: w1611 -> [w1630]
                        tunnel: [w1630] -> w1609 mode=indexing
                      }
                      n431 = call "WS1050 AD7747 READ.vi"("error in"=w1603, "Log (T)"=w1591, "DUT Mask Mode (All)"=WSVCAP_SHL_I2C_DUT_Mask_Mode_Enum."C2") -> ("error out"=w1601:errorcluster, "AD7747 Values"=w1599:string[][])  [unwired: 7 in]
                      n432 = for {
                        tunnel: w1599 -> [w1627] mode=indexing
                        tunnel: [w1628] -> w1600 mode=indexing
                        tunnel: w1601 -> [w1626]
                        tunnel: [w1626] -> w1598
                        n433 = Index Array(array=w1627, index=3) -> (element=w1628:string)
                      }
                      n434 = call "WS1050 AD7747 READ.vi"("error in"=w1598, "Log (T)"=w1591, "DUT Mask Mode (All)"=WSVCAP_SHL_I2C_DUT_Mask_Mode_Enum."C3") -> ("error out"=w1596:errorcluster, "AD7747 Values"=w1595:string[][])  [unwired: 7 in]
                      n435 = for {
                        tunnel: w1595 -> [w1623] mode=indexing
                        tunnel: [w1624] -> w1594 mode=indexing
                        tunnel: w1596 -> [w1622]
                        tunnel: [w1622] -> w1592
                        n436 = Index Array(array=w1623, index=5) -> (element=w1624:string)
                      }
                    }
                    n437 = local write "STATUS"("VSA Testing...." ("STATUS")) -> ()
                  }
                }
                n438 = Transpose 2D Array(2D array=w1546) -> (transposed array=w1544:string[][])
                n439 = Transpose 2D Array(2D array=w1545) -> (transposed array=w1543:string[][])
                n440 = Transpose 2D Array(2D array=w1542) -> (transposed array=w1541:string[][])
                n441 = Transpose 2D Array(2D array=w1539) -> (transposed array=w1538:string[][])
                n442 = call "WS1050_VSA_Convert_Data Updated.vi"("VSA_C3"=w1538, "WS1050/51"=w1526, "error in (no error)"=w1540, "VSA_C2"=w1541, "VSA_C1"=w1543, "Voltage"=w1544) -> ("error out"=w1537:errorcluster, "VSA_V3"=w1534:string[][], "VSA_V2"=w1535:string[][], "VSA_V1"=w1536:string[][])  [unwired: 2 in]
                "VSA_V1" <- w1536
                "VSA_V2" <- w1535
                "VSA_V3" <- w1534
                n443 = case shown="True" w1527 {
                  tunnel: w1556 -> [w1570 w1576]
                  tunnel: [w1570 w1575] -> w1555
                  tunnel: w1537 -> [w1569 w1574]
                  tunnel: [w1569 w1571] -> w1554
                  frame False {
                  }
                  frame True {
                    w1572 = u16 0 items=["Voltage", "Current"] ("Source Mode  (0: Voltage)")
                    n444 = call "Configure Output.vi"("Source Mode  (0: Voltage)"=w1572, "error in (no error)"=w1574, "Output Level (0)"=0.0, "VISA resource name"=w1576) -> ("error out"=w1571:errorcluster, "VISA resource name out"=w1575:refnum<visa-resource-name>)  [unwired: 6 in]
                  }
                }
                n445 = call "Delay T4.vi"("milliseconds to wait"=u32 50, "error in (no error)"=w1554) -> ("error out"=w1553:errorcluster)  [unwired: 9 in]
              }
              frame #6 {
                # "Handshake Check and EFuse Readback"
                n446 = Or(x=w1644, y=w1654) -> (x .or. y?=w1653:bool)
                n447 = Add(x=w1666, y=w1665) -> (x+y=w1652:u64)
                n448 = case shown="False" w1653 {
                  tunnel: w1679 -> [w1692 _]
                  tunnel: w1678 -> [w1691 w1696]
                  tunnel: [w1690 w1696] -> w1677
                  tunnel: w1676 -> [w1689 _]
                  tunnel: w1675 -> [w1688 _]
                  tunnel: w1674 -> [w1687 _]
                  tunnel: [w1683 w1695] -> w1673
                  tunnel: [w1682 w1695] -> w1668
                  tunnel: w1652 -> [w1681 _]
                  tunnel: w1659 -> [w1680 _]
                  frame False {
                    n449 = call "WS1050_16DUT_Handshake Check R1_Record All Regs Ver1.0.vi"("file path (use dialog)"=w1692, "Reg1_Bit Cntrl"="Reg1_Bit Cntrl", "File Name"=w1680, "SN"=w1687, "Loop"=w1681, "error"=w1691, "Lot #"=w1689, "Wafer #"=w1688) -> ("Pass/Fail"=→"EFuse Readback Status":bool[], "EFuse Read back"=w1682:string[], "Status"=w1683:string[], "error out"=w1690:errorcluster)  [unwired: 6 in, 2 out]
                    n450 = case shown="1, Default" w1681 {
                      tunnel: w1682 -> [w1693 w1694]
                      frame 0 {
                        "EFuse RB T0" <- w1693
                      }
                      frame 1, Default {
                        "Current EFuse Read back" <- w1694
                      }
                    }
                    n451 = local write "STATUS"("Hand Shake & EFuse Readback...." ("STATUS")) -> ()
                  }
                  frame True {
                    w1695 = string[] ["NA", "NA", "NA", "NA", "NA", "NA", "NA", "NA", "NA", "NA", "NA", "NA", "NA", "NA", "NA", "NA"] ("EFuse Read back")
                  }
                }
                n452 = Add(x=w1652, y=w1649) -> (x+y=w1650:u64)
                "TTime Completed" <- w1650
                n453 = Number To Engineering String(4:w1650) -> (0:w1664:string)  [unwired: 3 in]
                n454 = Build Array(w1663, w1661, w1660) -> (w1662:string[])
              }
              frame #7 {
                # "Save Data"
                n455 = Increment(x=w1707) -> (x+1=w1706:i32)
                n456 = local write "STATUS"("Saving Data...." ("STATUS")) -> ()
                n457 = Multiply(x=w1706, y=16) -> (x*y=w1701:i32)
                n458 = Path To String(path=w1711) -> (string=w1710:string)
                n459 = Bundle("Test Program"=w1744, "Comment"=w1743, "Data Out"=w1719, "Data Out"=w1717, "Data Out"=w1716, w1715, "Data Out"=w1714, "Data Out"=w1713, "string"=w1712, "Freq(Hz)"=w1699, "Brd #"=w1698) -> (w1718:T8)  [unwired: 1 in]
                n460 = case shown="True" "Debug" {
                  tunnel: w1701 -> [w1751 w1754]
                  tunnel: [w1751 w1752] -> w1700
                  frame False {
                  }
                  frame True {
                    n461 = Multiply(x=w1754, y="No of Rows\nFrom Spread Sheet") -> (x*y=w1752:i32)
                  }
                }
                n462 = call "WS1050_16 DUT SData ver1.3"("TMN DC\\CAP Data Log File Path"=w1711, "Lot#"=w1746, "Total Delta C1(pF)"=w1722, "VSA_V1"=w1731, "Wafer#"=w1742, "File Name"=w1704, "Total Delta C2(pF)"=w1721, "error in"=w1749, "TP/Comment"=w1718, "EFuse"=w1736, "Data Output C3"=w1724, "Temperature"=w1728, "VSA_V2"=w1732, "VPI C3"=w1726, "Data Output C1"=w1739, "VPI C2"=w1725, "SN"=w1747, "R/W Status"=w1745, "Cap Header"=w1727, "HD/Cycles Completed"=w1735, "Data Output C2"=w1723, "VSA_V3"=w1730, "Current"=w1738, "VPI C1"=w1737, "Total Delta C3(pF)"=w1720) -> ("error out"=w1748:errorcluster)  [unwired: 2 in]
                n463 = Concatenate Strings(w1710, "\\" ("string"), w1704, "_Multi Socket Data.csv" ("string")) -> (w1709:string)
              }
              frame #8 {
                n464 = case shown="True" "Plot Delta Cmin" {
                  tunnel: w1760 -> [w1775 w1791]
                  tunnel: [w1775 w1787] -> w1759
                  tunnel: w1758 -> [_ w1783]
                  tunnel: w1756 -> [_ w1781]
                  tunnel: w1755 -> [_ w1776]
                  frame False {
                  }
                  frame True {
                    n465 = String To Path(string=w1783) -> (path=w1782:path)
                    n466 = call "Delay T4.vi"("milliseconds to wait"=u32 50, "error in (no error)"=w1791) -> ("error out"=w1790:errorcluster)  [unwired: 9 in]
                    n467 = call "16DUT Plot Subvi Ver1.0.vi"("Plot"="Plot", "No of Rows"=w1781, "error in (no error)"=w1790, "WS1050/51"=w1776, "Bank"=enum16{"C1", "C2", "C3"}."C1", "file path (dialog if empty)"=w1782) -> ("error out"=w1785:errorcluster, "Delta C_Min Plot"=→"Min Plot_1":dbl[][])  [unwired: 4 in]
                    n468 = call "16DUT Plot Subvi Ver1.0.vi"("Plot"="Plot", "No of Rows"=w1781, "error in (no error)"=w1785, "WS1050/51"=w1776, "Bank"=enum16{"C1", "C2", "C3"}."C2", "file path (dialog if empty)"=w1782) -> ("error out"=w1786:errorcluster, "Delta C_Min Plot"=→"Min Plot_2":dbl[][])  [unwired: 4 in]
                    n469 = call "16DUT Plot Subvi Ver1.0.vi"("Plot"="Plot", "No of Rows"=w1781, "error in (no error)"=w1786, "WS1050/51"=w1776, "Bank"=enum16{"C1", "C2", "C3"}."C3", "file path (dialog if empty)"=w1782) -> ("error out"=w1787:errorcluster, "Delta C_Min Plot"=→"Min Plot_3":dbl[][])  [unwired: 4 in]
                  }
                }
                n470 = Get Date/Time In Seconds() -> (seconds since 1Jan1904=w1768:timestamp)
                n471 = Get Date/Time String(seconds (now)=w1768, want seconds? (F)=TRUE) -> (date string=→"date string":string, time string=→"Previous Time":string)  [unwired: 1 in]
                n472 = Greater Or Equal?(x=w1764, y="TTF Completed") -> (x >= y?=w1763:bool)
                n473 = Greater Or Equal?(x=w1765, y="Set HD/Cycle \nto Complete") -> (x >= y?=w1772:bool)
                "No of HD/Cycle\nCompleted" <- w1765
              }
            }
            n474 = Increment(x=w521) -> (x+1=→"Loop \ncompleted":i32)
            n475 = call "Delay T4.vi"("milliseconds to wait"=u32 50, "error in (no error)"=w408) -> ("error out"=w409:errorcluster)  [unwired: 9 in]
            n476 = Compound Arithmetic op=OR(w593, w491, w517) -> (w530:bool)
          }
          "Total Time" <- w355
          n477 = Increment(x=w353) -> (x+1=→"Running Loops":i32)
          n478 = local write "No of HD/Cycle\nCompleted"(u64 0 ("No of HD/Cycle\nCompleted")) -> ()
          n479 = Unbundle By Name(w345) -> ("status"=w359:bool)
          n480 = Compound Arithmetic op=OR(w359, w351, w350) -> (w341:bool)
        }
        n481 = for {
          tunnel: w271 -> [w1802]
          tunnel: w301 -> [w1801]
          tunnel: w302 -> [w1798] mode=indexing
          tunnel: [w1793] -> w269
          tunnel: [w1797] -> w300
          n482 = call "E3631A_Voltage Controller.vi"("VISA resource name"=w1801, "Channel Controller"=w1798, "Voltage 1"=0.0, "Voltage 2"=3.3, "error in (no error)"=w1802, "Voltage 3"=-3.3) -> ("VISA resource name out"=w1797:refnum<visa-resource-name>, "error out"=w1794:errorcluster)  [unwired: 8 in]
          n483 = call "Delay T4.vi"("milliseconds to wait"=u32 100, "error in (no error)"=w1794) -> ("error out"=w1793:errorcluster)  [unwired: 9 in]
        }
        n484 = VISA Write(VISA resource name=w291, write buffer="SOUR:FUNC VOLT;VOLT:MODE FIX;RANG 100;LEV 0.0;:SENS:FUNC \"CURR\";CURR:PROT 60E-3;RANG 100E-3;:OUTP ON", error in (no error)=w271) -> (VISA resource name out=w289:refnum<visa-resource-name>, error out=w270:errorcluster)  [unwired: 1 out]
        n485 = Merge Errors(w269, w270) -> (w290:errorcluster)
      }
      frame True {
      }
    }
    n486 = local write "stop During HD/Cycles"(w60) -> ()
    n487 = Unbundle By Name(w61) -> ("status"=w81:bool)
    n488 = Or(x=w81, y=w70) -> (x .or. y?=w80:bool)
    n489 = Wait Until Next ms Multiple(millisecond multiple=u32 100) -> ()  [unwired: 1 out]
    "STATUS" <- "Idle...." ("STATUS")
  }
  "Ke2000 Out" <- w21
  "PS1 Out" <- w20
  n490 = local write "stop During HD/Cycles"(w6) -> ()
  n491 = local write "stop"(w6) -> ()
  n492 = case shown="True" w18 {
    tunnel: [w1819 w1821] -> w1
    tunnel: w12 -> [w1819 w1820]
    frame False {
    }
    frame True {
      n493 = flat-sequence {
        tunnel: w1820 -> [w1824]
        tunnel: [w1823] -> w1821
        frame #0 {
          n494 = local write "Online"(FALSE ("Online")) -> ()
          n495 = call "WSVCAP SHL Host TL Close.vi"("error in"=w1824) -> ("error out"=w1823:errorcluster)  [unwired: 14 in]
        }
      }
    }
  }
  "error out" <- w1
  n496 = VISA Write(VISA resource name=w13, write buffer="SOUR:FUNC VOLT;VOLT:MODE FIX;RANG 100;LEV 0.0;:SENS:FUNC \"CURR\";CURR:PROT 60E-3;RANG 100E-3;:OUTP OFF", error in (no error)=w12) -> (VISA resource name out=→"VISA resource name out":refnum<visa-resource-name>, error out=→"error out 2":errorcluster)  [unwired: 1 out]
